vi "Lockin-4461 -Patrick -State.vi"(10 "IV Curve Mode":bool, 11 "Channels: AO":T6={"AO amp (V)"=[0.01, 0.0, 0.0, 0.0, 0.0, 0.0, 0.0, 0.0], "AO DC (V)"=[0.0, 0.0, 0.0, 0.0, 0.0, 0.0, 0.0, 0.0], "AO f (Hz)"=[13.1, 13.0, 13.0, 13.0, 13.0, 13.0, 13.0, 13.0], "AO phi (deg)"=[0.0, 0.0, 0.0, 0.0, 0.0, 0.0, 0.0, 0.0], "function"=[enum."Sine Wave", enum."Sine Wave", enum."Sine Wave", enum."Sine Wave", enum."Sine Wave", enum."Sine Wave", enum."Sine Wave", enum."Sine Wave"]} {"AO f (Hz)" min=0.001 max=10000.0; "AO DC (V)" format="%#_6p"; "AO amp (V)" format="%#_6p"}) -> ()   [LabVIEW 2016]
uses:
  Typedefs/AO-cluster.ctl
  Typedefs/AO_Amp-array.ctl
  Typedefs/AO_DC-array.ctl
  Typedefs/AO_f-array.ctl
  Typedefs/AO_phi-array.ctl
  Typedefs/Function-array.ctl
  Typedefs/Function-enum.ctl
  Typedefs/REF-cluster.ctl
  Typedefs/REF_f-array.ctl
  Typedefs/REF_phi-array.ctl
  Typedefs/AO.config-cluster.ctl
  Typedefs/AI.config-cluster.ctl
  Typedefs/AI.coupling-enum.ctl
  <vilib>/Analysis/4window.llb/windowTd.ctl
  <vilib>/measure/maspectr.llb/Power Spectrum and PSD Export Mode.ctl
  <vilib>/Utility/error.llb/DialogType.ctl
  <vilib>/Analysis/baseanly.llb/Mean (DBL).vi
  <userlib>/_OpenG.lib/array/array.llb/Empty 1D Array (Variant)__ogtk.vi
  <vilib>/Platform/browser.llb/Open URL in Default Browser (string).vi
  <userlib>/_OpenG.lib/error/error.llb/Filter Error Codes (Array)__ogtk.vi
  <userlib>/_OpenG.lib/array/array.llb/Empty 1D Array (DBL)__ogtk.vi
  <vilib>/measure/maspectr.llb/FFT Power Spectrum and PSD for N Chan.vi
  <vilib>/Waveform/WDTOps.llb/WDT Waveform to XY Pairs DBL.vi
  <vilib>/measure/NI_MAPro.lvlib
  <vilib>/Analysis/NI_AALBase.lvlib
  <vilib>/Utility/config.llb/NI_LVConfig.lvlib
  <vilib>/Analysis/NI_AALPro.lvlib
panel:
  in  "Tab Control 3":enum32{"Page 1"}(tab)
  in  "Bug":bool
  in  "Trigger":bool
  in  "Notes":string
  in  "Path":path=path "C:/Data/lockin"
  in  "EXIT":bool
  in  "RESET":bool
  in  "Save Data":bool
  out "X or R":dbl=-1.5674776385045113e-05 caption="X or R: Current (A) or Voltage (V)" format="%#.3p"
  out "Y or Theta":dbl=0.0006969030734106954 caption="Y or Theta: Current (A) or Voltage (V)" format="%.3p"
  in  "Display":enum16{"X and Y", "R and Theta"}(ring)
  in  "Channel":dbl min=0.0 max=7.0 step=1.0
  in  "Remote Mode":bool
  out "time and date":string="18:32:49.6   2017-07-28"
  out "DAQ mode string":string="None"
  out "time since trigger":dbl
  in  "mean":dbl[](array[numeric])=[0.0020212134088697844, -0.0038683061420776745, -0.0017577206979397751, -6.13137174522516e-05, -0.0025607955795279433, -0.0022408587829792284, 0.0003178164150233449, -0.0028469064949645513]
  in  "Tab Control 2":T1(tab)
  in  "Output signals?":bool=TRUE
  out "Signals Graph":waveform(dbl)[](graph)
  out "Reference Graph":waveform(dbl)[](graph)
  in  "decimate graph":i32=1
  in  "Display n?":bool=TRUE
  out "Display X (or R)":waveform(dbl)[](graph)=[{"t0"=timestamp(3584125969.6966953 s since 1904-01-01), "dt"=1.0, "Y"=[-1.5674776385045113e-05]}, {"t0"=timestamp(3584125969.6966953 s since 1904-01-01), "dt"=1.0, "Y"=[-8.70673776379909e-05]}, {"t0"=timestamp(3584125969.6966953 s since 1904-01-01), "dt"=1.0, "Y"=[-2.1693329226816633e-05]}, {"t0"=timestamp(3584125969.6966953 s since 1904-01-01), "dt"=1.0, "Y"=[-8.095080721838651e-05]}, {"t0"=timestamp(3584125969.6966953 s since 1904-01-01), "dt"=1.0, "Y"=[-9.220716518858501e-05]}, {"t0"=timestamp(3584125969.6966953 s since 1904-01-01), "dt"=1.0, "Y"=[-8.659365208742522e-05]}, {"t0"=timestamp(3584125969.6966953 s since 1904-01-01), "dt"=1.0, "Y"=[-0.0001111506406949471]}, {"t0"=timestamp(3584125969.6966953 s since 1904-01-01), "dt"=1.0, "Y"=[2.9050024564198337e-06]}]
  out "Display Y (or Theta)":waveform(dbl)[](graph)=[{"t0"=timestamp(3584125969.6966953 s since 1904-01-01), "dt"=1.0, "Y"=[0.0006969030734106954]}, {"t0"=timestamp(3584125969.6966953 s since 1904-01-01), "dt"=1.0, "Y"=[5.552511744346625e-05]}, {"t0"=timestamp(3584125969.6966953 s since 1904-01-01), "dt"=1.0, "Y"=[0.0001768914126496754]}, {"t0"=timestamp(3584125969.6966953 s since 1904-01-01), "dt"=1.0, "Y"=[3.781436113329896e-05]}, {"t0"=timestamp(3584125969.6966953 s since 1904-01-01), "dt"=1.0, "Y"=[-0.00011680861026454419]}, {"t0"=timestamp(3584125969.6966953 s since 1904-01-01), "dt"=1.0, "Y"=[-9.443651807610673e-05]}, {"t0"=timestamp(3584125969.6966953 s since 1904-01-01), "dt"=1.0, "Y"=[8.143626032195178e-05]}, {"t0"=timestamp(3584125969.6966953 s since 1904-01-01), "dt"=1.0, "Y"=[-0.0003099144140816687]}]
  out "XY Graph":cluster{dbl[], dbl[]}[](graph)=[{[0.0, -1.5674776385045113e-05], [0.0, 0.0006969030734106954]}, {[0.0, -8.70673776379909e-05], [0.0, 5.552511744346625e-05]}, {[0.0, -2.1693329226816633e-05], [0.0, 0.0001768914126496754]}, {[0.0, -8.095080721838651e-05], [0.0, 3.781436113329896e-05]}, {[0.0, -9.220716518858501e-05], [0.0, -0.00011680861026454419]}, {[0.0, -8.659365208742522e-05], [0.0, -9.443651807610673e-05]}, {[0.0, -0.0001111506406949471], [0.0, 8.143626032195178e-05]}, {[0.0, 2.9050024564198337e-06], [0.0, -0.0003099144140816687]}]
  out "Results\n(X, Y, R, Theta, mean)":dbl[][](array[numeric])=[[-1.5674776385045113e-05, 0.0006969030734106954, 0.000697079330022053, 91.28848209297018, 0.0020212134088697844], [-8.70673776379909e-05, 5.552511744346625e-05, 0.00010326551658645415, 147.4732893773882, -0.0038683061420776745], [-2.1693329226816633e-05, 0.0001768914126496754, 0.000178216644570985, 96.99163795294015, -0.0017577206979397751], [-8.095080721838651e-05, 3.781436113329896e-05, 8.934740677394016e-05, 154.96142087956403, -6.13137174522516e-05], [-9.220716518858501e-05, -0.00011680861026454419, 0.00014881670855132224, -128.28709336414173, -0.0025607955795279433], [-8.659365208742522e-05, -9.443651807610673e-05, 0.00012812773520271432, -132.51929584201363, -0.0022408587829792284], [-0.0001111506406949471, 8.143626032195178e-05, 0.0001377908902000489, 143.77104596378203, 0.0003178164150233449], [2.9050024564198337e-06, -0.0003099144140816687, 0.0003099280288951869, -89.46295009810324, -0.0028469064949645513]] format="%#_3p"
  out "PS Chart":dbl[][](graph)=[[-1105.6899114588311, -1143.9798102016132, -1120.3260349628486, -1104.2479960602075, -1135.3349531393583, -1128.801716551488, -1154.426424169608, -1125.1608260528487]]
  out "PS dB":cluster{"f0":dbl, "df":dbl, "magnitude":dbl[]}[](graph)
  in  "window":T2=1 items=["Rectangle"=0, "Hanning"=1, "Hamming"=2, "Blackman-Harris"=3, "Exact Blackman"=4, "Blackman"=5, "Flat Top"=6, "4 Term B-Harris "=7, "7 Term B-Harris"=8, "Low Sidelobe"=9, "Blackman Nuttall"=11, "Triangle"=30, "Bartlett-Hanning"=31, "Bohman"=32, "Parzen"=33, "Welch"=34, "Kaiser"=60, "Dolph-Chebyshev"=61, "Gaussian"=62]
  in  "averaging parameters":T3={"averaging mode"=enum."RMS averaging", "weighting mode"=enum."Exponential", "number of averages"=10} {"number of averages" min=1}
  in  "restart averaging (F)":bool
  in  "export mode":T4 items=["Power Spectrum", "Power Spectral Density"]
  in  "window parameter":dbl=nan
  out "averages\ncompleted":dbl=2.0
  out "averaging done":bool
  in  "Tab Control":T5(tab)
  in  "...............reset REF":bool
  in  "............zero offset":bool
  in  "....measure offset":bool
  in  "............all  f same":bool
  in  "..........reset signal":bool
  in  "60 Hz prefilter":bool
  in  "LP prefilter":bool
  in  "LP cutoff (Hz)":dbl=30.0
  in  "Channels: Lockin":T13={"REF f (Hz)"=[13.0], "REF phi (deg)"=[0.0, 0.0, 0.0, 0.0, 0.0, 0.0, 0.0, 0.0]} {"REF phi (deg)" format="%#_3g"}
  in  "D":dbl=0.019999999999999997 format="%.2f"
  in  "I":dbl=0.6 format="%.2f"
  in  "P":dbl=0.5 format="%.2f"
  in  "autophase?\n(experimental)":bool
  out "filter fC (Hz)":dbl=0.5305164769729844
  in  "TC (s)":dbl=0.3 format="%#_6p"
  in  "order":i32=2
  in  "save config":bool
  in  "load config":bool
  in  "Instrument":u16(ring) items=["SIMULATE", "CF900", "DR200", "MNK", "PPMS1", "PPMS2", "THz1", "THz2"]
  in  "AO Configuration":T16[](array[typedef])
  in  "AI Configuration":T17[](array[typedef])
  in  "#s":i32=15630
  in  "Fs":i32=204753
  in  "auto size":bool=TRUE
  in  "decimating factor":i32=1
  in  "AI Buffer Size (S)":i32=100
  out "dt":dbl=4.883933324542254e-06 format="%#_6p"
  in  "frequency multiplier":dbl=100000.0 format="%#_13g"
  out "sampling info":cluster{"Fs":i32, "#s":i32}={"Fs"=4000, "#s"=10000}
  in  "DAQ Type":enum16{"None", "USB 4431", "PXI 446x"}(ring)
  in  "Amplifiers":enum16{"None", "Krohn Hite", "Femto"}(ring)
  out "Current State":string="Exit"
  out "State History":string="4461: PHASE\r4461: LOCKIN\rMacro: Continuous\r4461: READ WRITE\r4461: FILTER\r4461: PHASE\r4461: LOCKIN\r4461: STOP TASKS\rMacro: Exit\rData: Cleanup\rExit"
  in  "offsets":dbl[](array[numeric])=[0.0, 0.0, 0.0, 0.0, 0.0, 0.0, 0.0, 0.0] format="%#.2p"
  in  "Gain":dbl[](array[numeric])=[1.0, 1.0, 1.0, 1.0, 1.0, 1.0, 1.0, 1.0]
  out "phase log":dbl[](array[numeric])=[0.0, 272.06106870229246, 272.06106870229246, 272.06106870229246, 272.06106870229246, 272.06106870229246, 272.06106870229246, 272.06106870229246] format="%.1f"
  out "AI tasks":i32
  out "AO tasks":i32
  out "error":errorcluster
  in  "Check Calibration":bool
  in  "Self Calibrate":bool
  out "Cal Info":T19(array[cluster])
  # "´"
  # "Multichannel Lockin v2017/10/09 v2.4.4"
  # "plot 0    = AI0 f0\nplot 1    = Ai1 f0\n...\nplot N-1  = AIN f0\n\nplot N    = AI0 f1\nplot N+1  = AI1 f1\n..."
  # "AO Settings"
  # "Lockin Settings"
  # "prefilters"
  # "lockin filter"
  # "autophase"
  # "0"
  # "1"
  # "2"
  # "3"
  # "4"
  # "5"
  # "6"
  # "7"
  # "configuration"
  # "sampling"
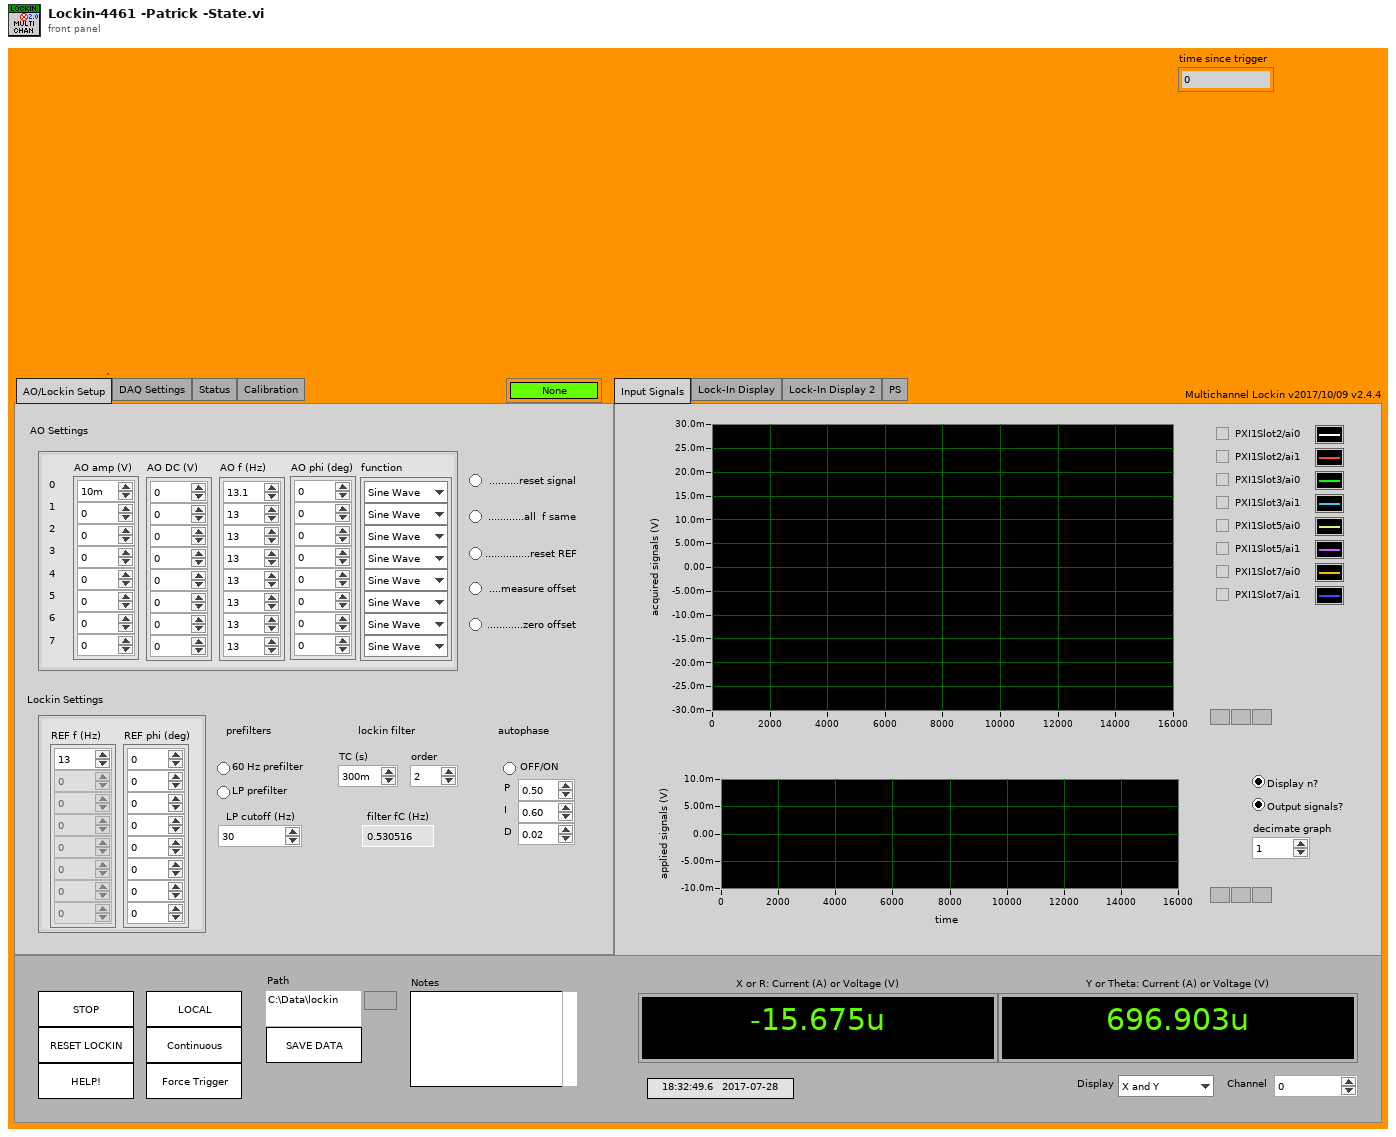
[diagram p1: front panel]
types:
  T1 = enum32{"Input Signals", "Lock-In Display", "Lock-In Display 2", "PS"}
  T2 = typedef "NI_AALPro.lvlib/windowTd.ctl" = u32
  T3 = cluster{"averaging mode":enum16{"No averaging", "Vector averaging", "RMS averaging", "Peak hold"}, "weighting mode":enum16{"Linear", "Exponential"}, "number of averages":u32}
  T4 = typedef "NI_MAPro.lvlib/Power Spectrum and PSD Export Mode.ctl" = u16
  T5 = enum32{"AO/Lockin Setup", "DAQ Settings", "Status", "Calibration"}
  T6 = typedef "AO-cluster.ctl" = cluster{"AO amp (V)":T7, "AO DC (V)":T8, "AO f (Hz)":T9, "AO phi (deg)":T10, "function":T11}
  T7 = typedef "AO_Amp-array.ctl" = dbl[]
  T8 = typedef "AO_DC-array.ctl" = dbl[]
  T9 = typedef "AO_f-array.ctl" = dbl[]
  T10 = typedef "AO_phi-array.ctl" = dbl[]
  T11 = typedef "Function-array.ctl" = T12[]
  T12 = typedef "Function-enum.ctl" = enum16{"Sine Wave", "Triangle Wave", "Square Wave", "Sawtooth Wave"}
  T13 = typedef "REF-cluster.ctl" = cluster{"REF f (Hz)":T14, "REF phi (deg)":T15}
  T14 = typedef "REF_f-array.ctl" = dbl[]
  T15 = typedef "REF_phi-array.ctl" = dbl[]
  T16 = typedef "AO.config-cluster.ctl" = cluster{"Output physical channels":tag, "AO. Max":dbl, "AO.Min":dbl}
  T17 = typedef "AI.config-cluster.ctl" = cluster{"AI.Coupling":T18, "AI.Max":dbl, "AI.Min":dbl, "Input physical channels":tag}
  T18 = typedef "AI.coupling-enum.ctl" = enum16{"AC", "DC", "GND"}
  T19 = cluster{tag, "SelfCal.LastDate/Time":timestamp, "SelfCal.LastTemp":dbl, "DevTemp":dbl, "calibration due?":bool}[]
  T20 = enum32{"invalid app kind", "Development System", "Run Time System", "Student Edition", "Embedded LabVIEW", "Evaluation", "Custom"}
  T21 = enum32{"Invalid", "Standard", "Closed", "Hidden", "Minimized", "Maximized"}
  T22 = cluster{"REF f (Hz)":dbl[], "REF phi (deg)":dbl[]}
  T23 = cluster{"AO amp (V)":dbl[], "AO DC (V)":dbl[], "AO f (Hz)":dbl[], "AO phi (deg)":dbl[], "function":enum16{"Sine Wave", "Triangle Wave", "Square Wave", "Sawtooth Wave"}[]}
  T24 = cluster{"Core":cluster{"Current VI Reference":refnum<vi>, "Close Panel on Exit?":bool}, "Error":bool, "Your string data":string, "AI task":refnum<k21>[], "AO task":refnum<k21>[], "Input Signals":waveform(dbl)[], "Ouput Signals":waveform(dbl)[], "REF":waveform(dbl)[], "sampling info":cluster{"Fs":dbl, "#s":dbl}, "Tasks":string[], "to":i32}
  T25 = typedef "DialogType.ctl" = u16
  T26 = cluster{"Current VI Reference":refnum<vi>, "Close Panel on Exit?":bool}
  T27 = cluster{"Output physical channels":tag, "AO. Max":dbl, "AO.Min":dbl}[]
  T28 = cluster{"AI.Coupling":enum16{"AC", "DC", "GND"}, "AI.Max":dbl, "AI.Min":dbl, "Input physical channels":tag}[]
  T29 = cluster{tag, "SelfCal.LastDate/Time":timestamp, "SelfCal.LastTemp":dbl, "DevTemp":dbl, "recalibrate?":bool}[]
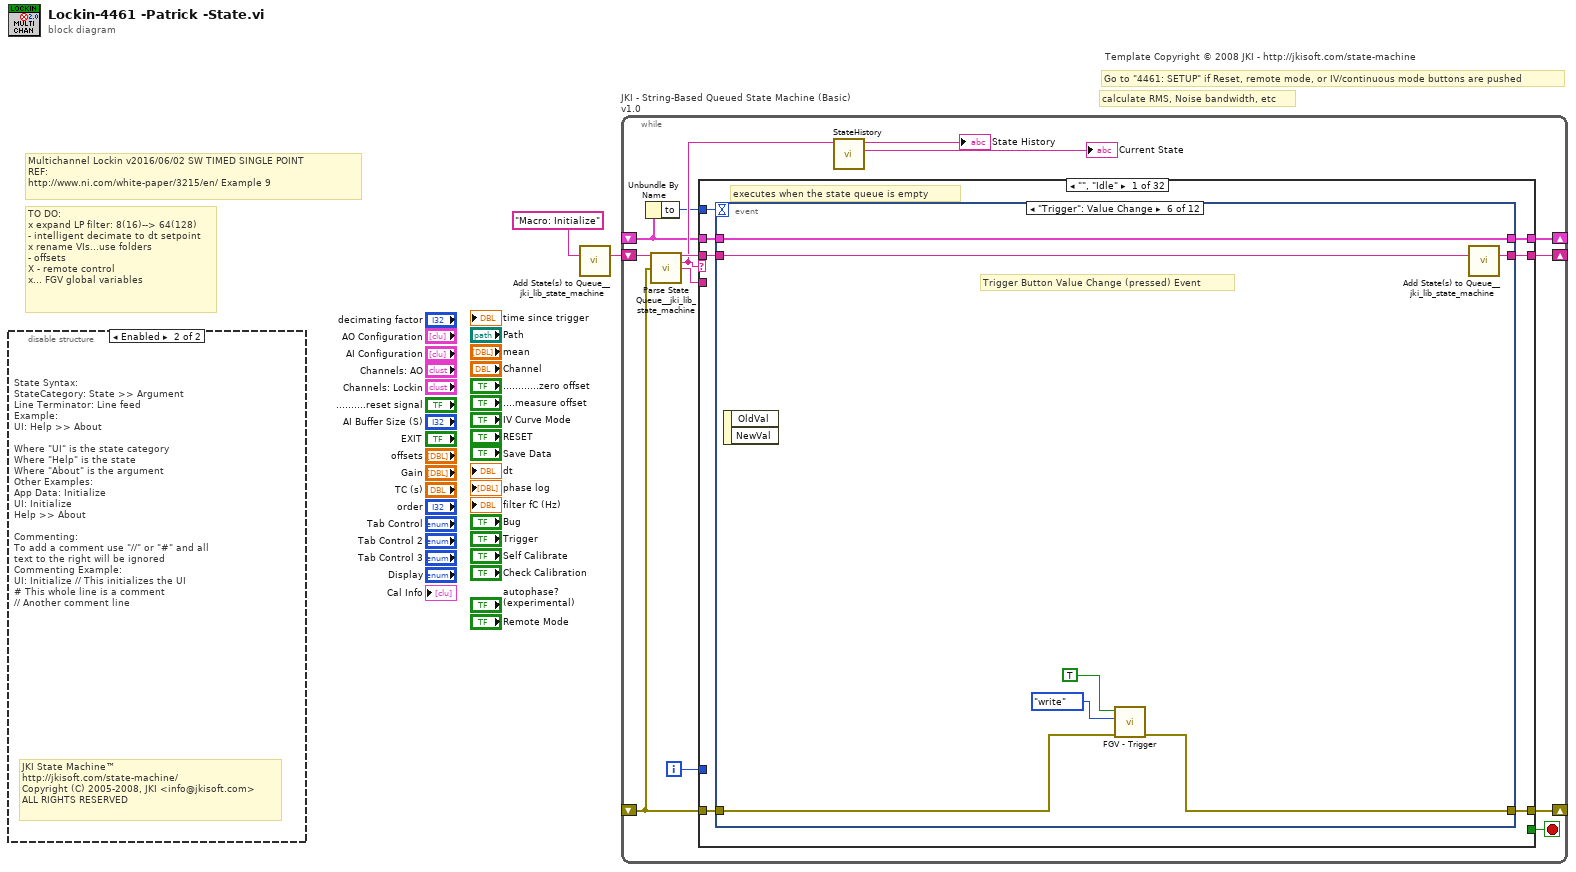
[diagram p0: block diagram]
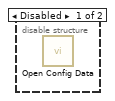
[diagram p2: hidden frame]
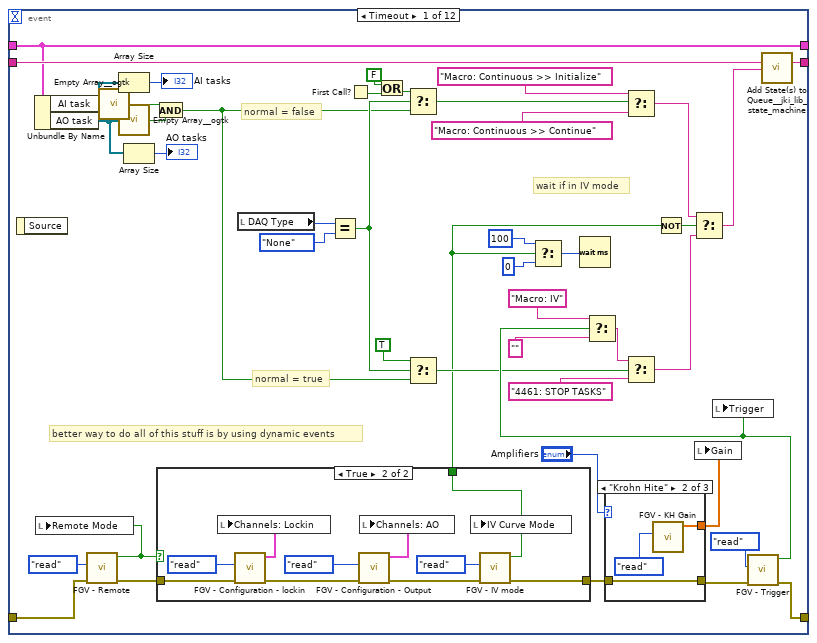
[diagram p3: hidden frame]
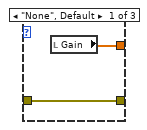
[diagram p4: hidden frame]
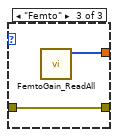
[diagram p5: hidden frame]
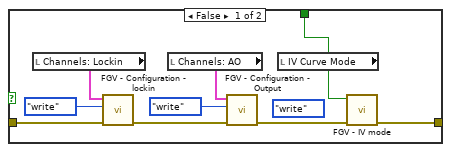
[diagram p6: hidden frame]
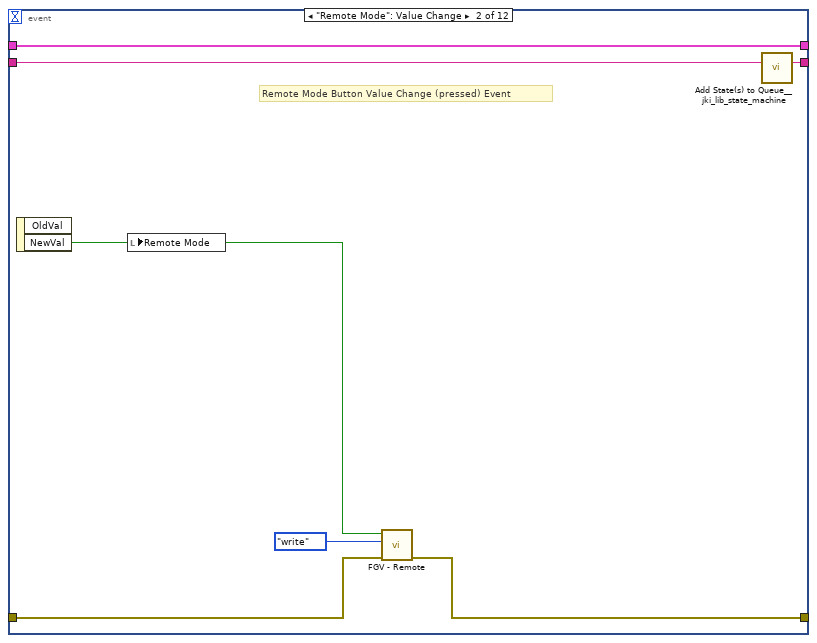
[diagram p7: hidden frame]
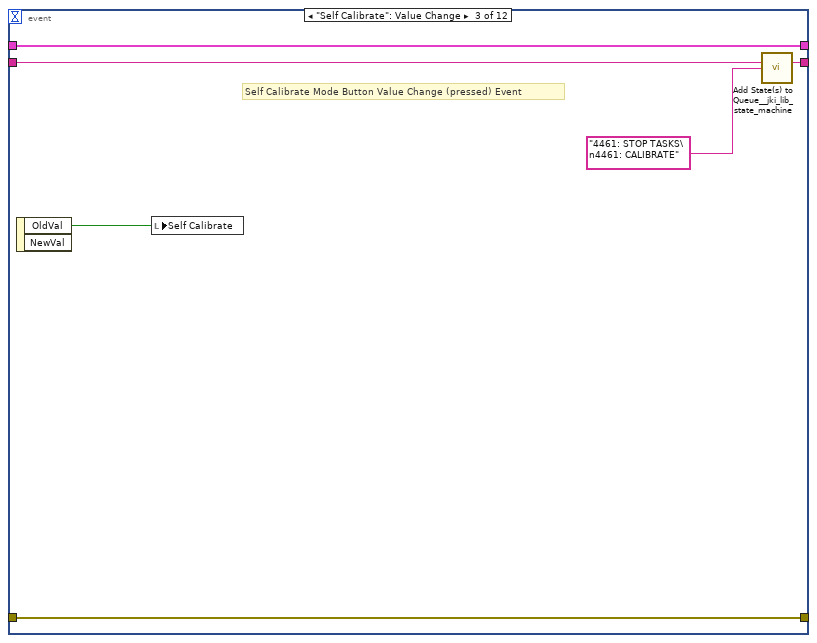
[diagram p8: hidden frame]
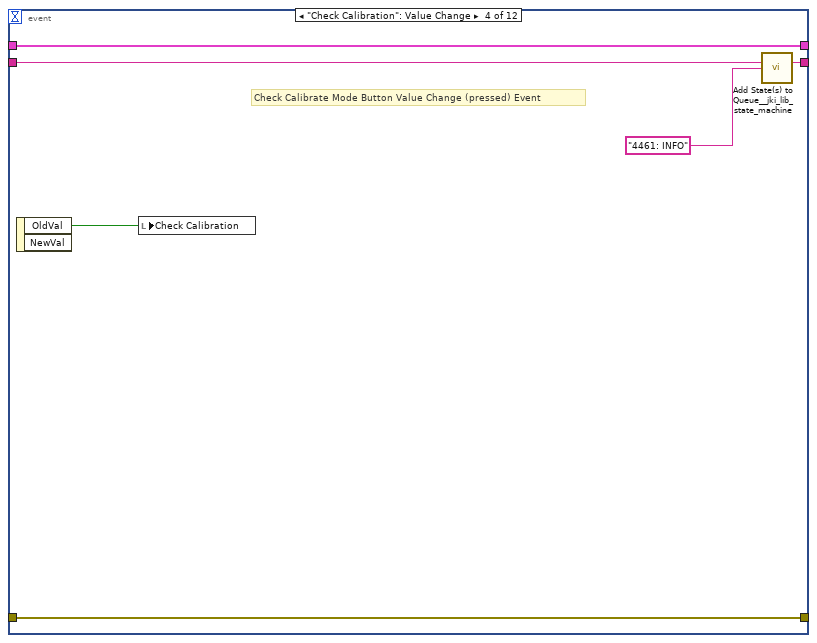
[diagram p9: hidden frame]
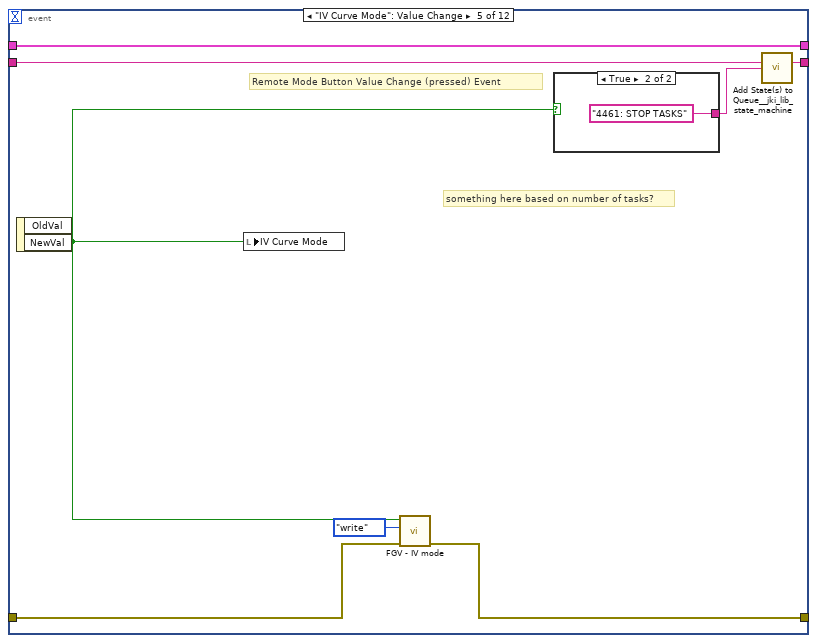
[diagram p10: hidden frame]
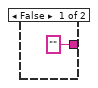
[diagram p11: hidden frame]
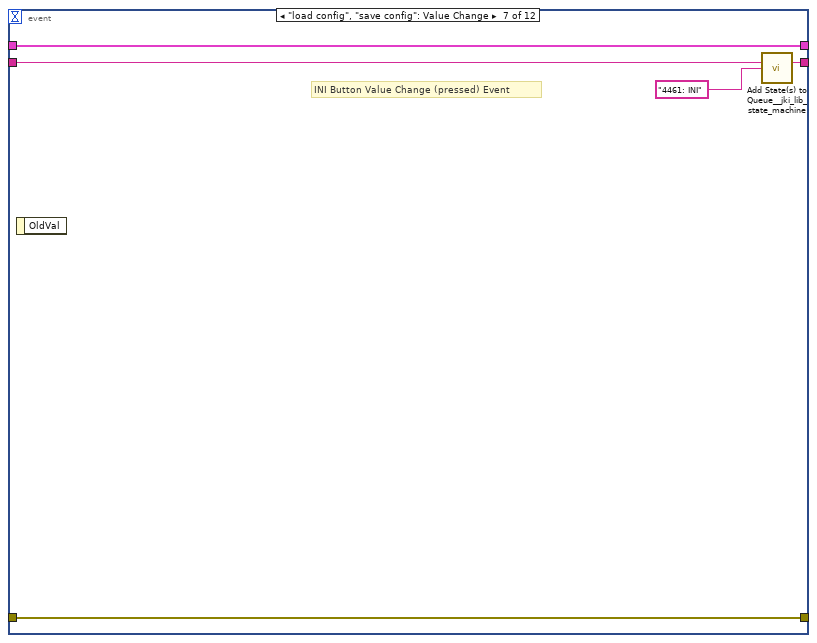
[diagram p12: hidden frame]
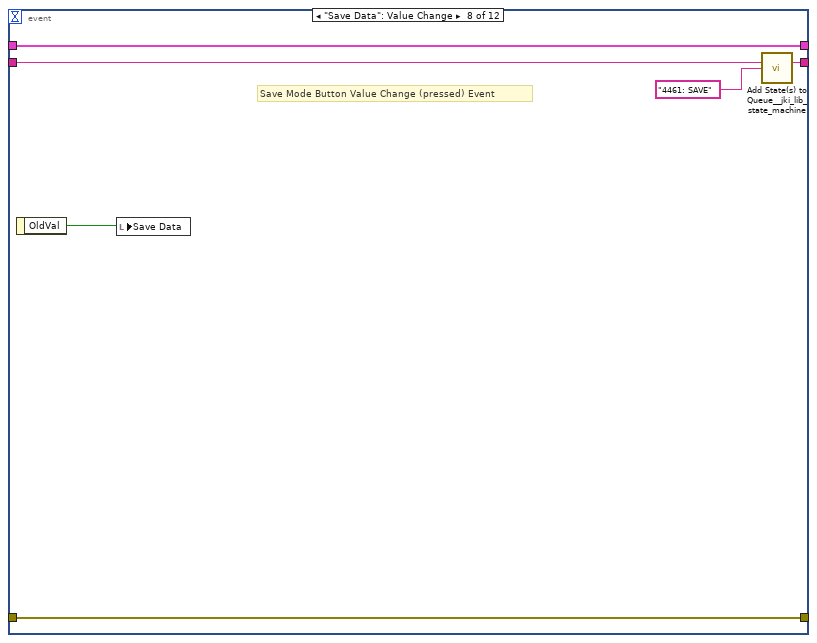
[diagram p13: hidden frame]
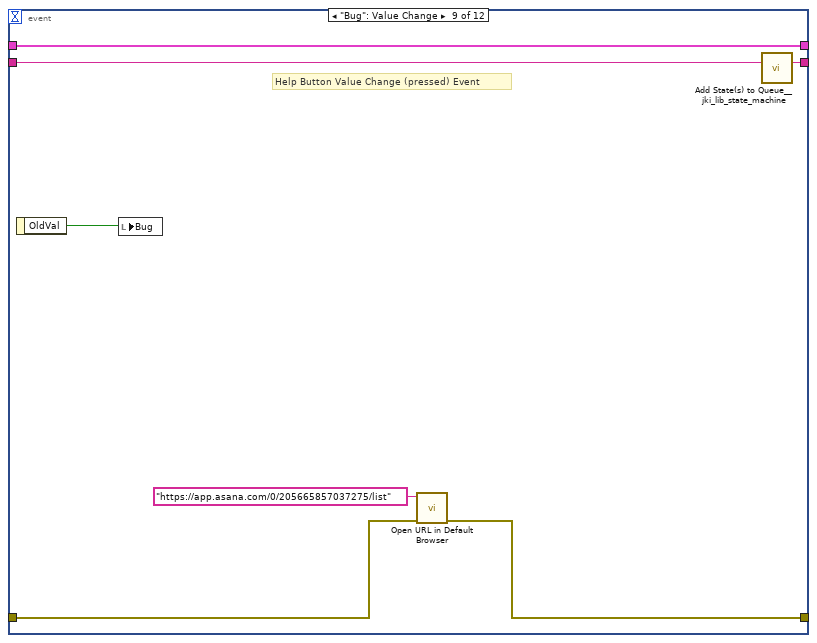
[diagram p14: hidden frame]
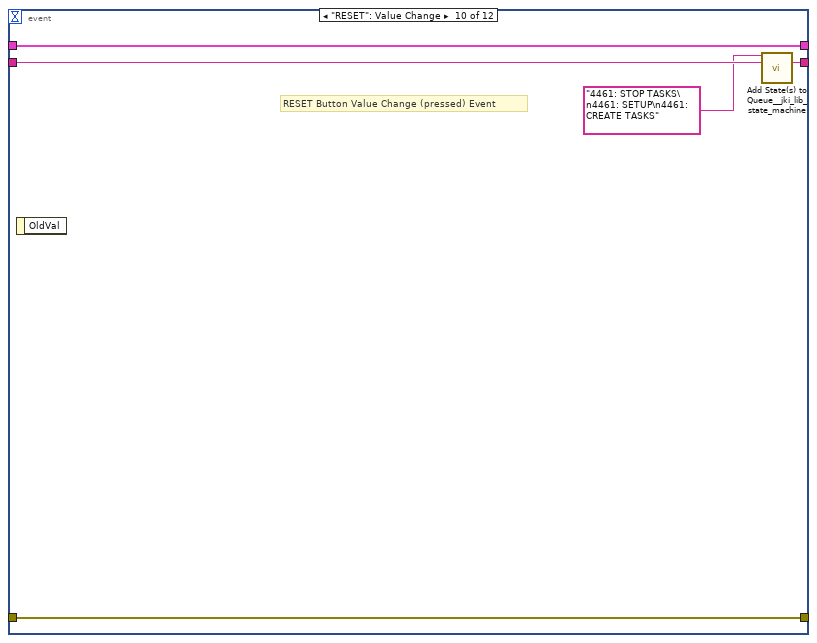
[diagram p15: hidden frame]
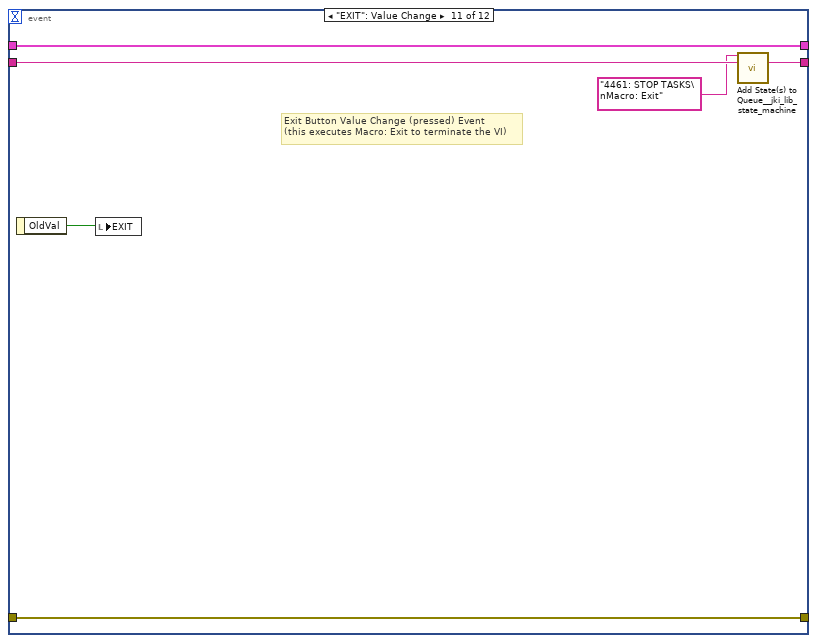
[diagram p16: hidden frame]
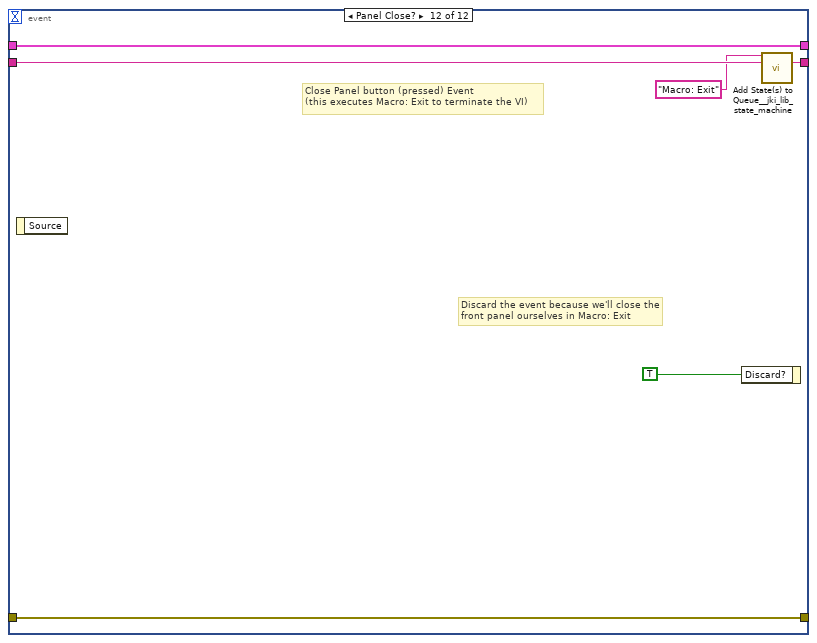
[diagram p17: hidden frame]
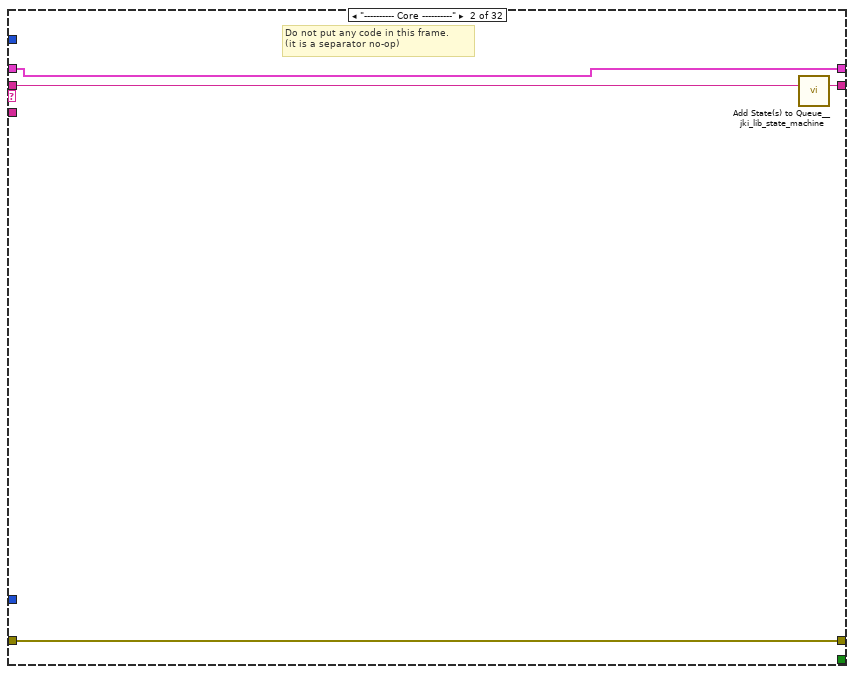
[diagram p18: hidden frame]
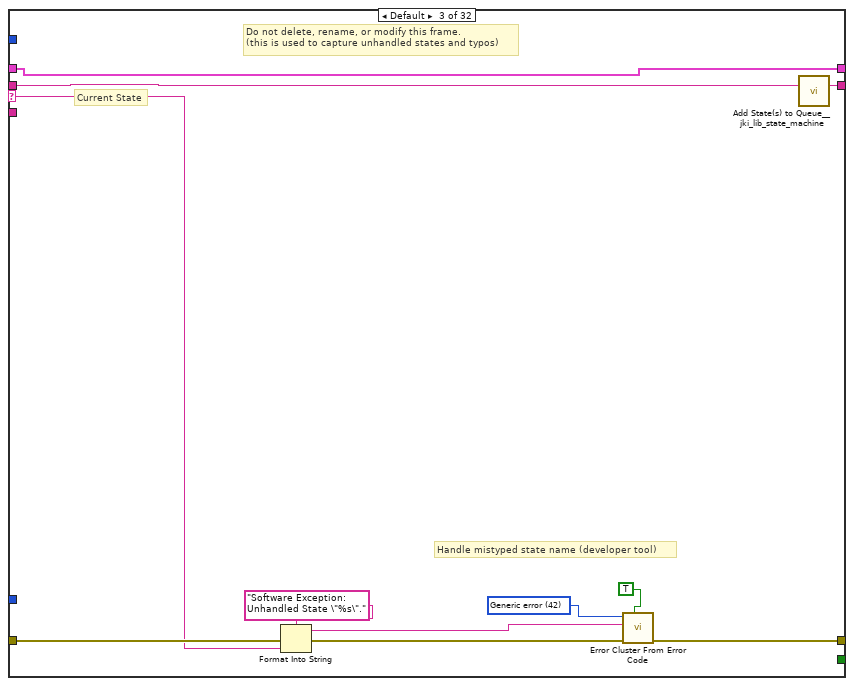
[diagram p19: hidden frame]
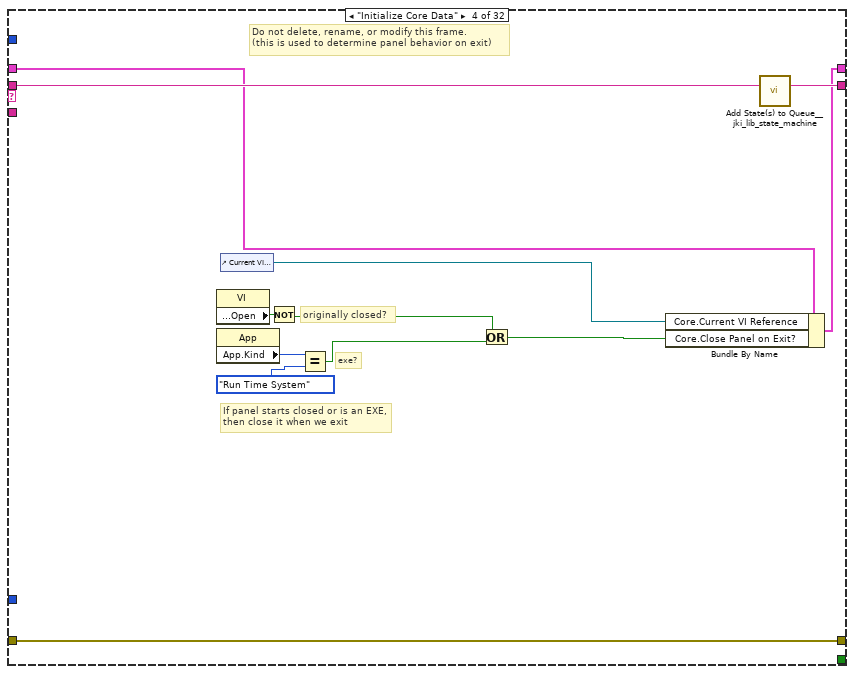
[diagram p20: hidden frame]
diagram:
  # "calculate RMS, Noise bandwidth, etc"
  # "Template Copyright © 2008 JKI - http://jkisoft.com/state-machine"
  # "Go to \"4461: SETUP\" if Reset, remote mode, or IV/continuous mode buttons are pushed"
  # "Multichannel Lockin v2016/06/02 SW TIMED SINGLE POINT\nREF:\nhttp://www.ni.com/white-paper/3215/en/ Example 9"
  # "TO DO:\nx expand LP filter: 8(16)--> 64(128)\n- intelligent decimate to dt setpoint\nx rename VIs...use folders\n- offsets\nX - remote control\nx... FGV global variables"
  n1 = disable-structure shown="Enabled" {
    frame Disabled {
      n2 = call <vilib>:"Open Config Data.vi"() -> ()  [unwired: 9 in, 3 out]
    }
    frame Enabled {
      # "JKI State Machine™\nhttp://jkisoft.com/state-machine/\nCopyright (C) 2005-2008, JKI <info@jkisoft.com>\nALL RIGHTS RESERVED"
      # "State Syntax:\nStateCategory: State >> Argument\nLine Terminator: Line feed\nExample:\nUI: Help >> About\n\nWhere \"UI\" is the state category\nWhere \"Help\" is the state\nWhere \"About\" is the argument\nOther Examples:\nApp Data: Initialize\nUI: Initialize\nHelp >> About\n\nCommenting:\nTo add a comment use \"//\" or \"#\" and all text to the right will be ignored\nCommenting Example:\nUI: Initialize // This initializes the UI\n# This whole line is a comment\n// Another comment line"
    }
  }
  n3 = call <vilib>:"Add State(s) to Queue__jki_lib_state_machine.vi"("State(s) in (\"\")"="Macro: Initialize") -> ("States Out"=w2:string)  [unwired: 14 in]
  n4 = while "JKI - String-Based Queued State Machine (Basic) v1.0" {
    shift-right: [w7] -> _
    shift-left: _ -> [w4]
    shift-right: [w15] -> _
    shift-left: _ -> [w8]
    shift-right: [w14] -> _
    shift-left: w2 -> [w9]
    i -> [w11]
    stop <- w13 stop-if-true
    n5 = Unbundle By Name(w4) -> ("to"=w3:i32)
    n6 = call <vilib>:"Parse State Queue__jki_lib_state_machine.vi"("State Queue"=w9, "Error In (no error)"=w8) -> ("Remaining States"=w12:string, "Current State"=w5:string, "Arguments"=w16:string)  [unwired: 11 in]
    n7 = case shown="\"\", \"Idle\"" w5 {
      selector: w5 -> [_ _ w169 _ _ _ _ _ _ _ _ _ _ _ _ _ _ _ _ _ _ _ _ _ _ _ _ _ _ _ _ _]
      tunnel: w16 -> [_ _ _ _ _ _ _ _ _ _ _ w256 w267 _ _ _ w309 _ _ _ _ _ _ _ _ _ _ _ _ _ _ _]
      tunnel: w4 -> [w21 w165 w171 w182 w197 w209 w212 _ w231 w237 w252 w255 w266 w294 w298 w303 w310 w316 w327 w336 w364 w414 w423 w436 w514 w565 w621 w686 w717 w765 w793 w841]
      tunnel: [w20 w166 w175 w188 errorcluster {"status"=FALSE, "code"=0, "source"=""} ("error out") w208 w213 w227 w232 w238 w246 w257 w265 w295 w300 w305 w311 w324 w328 w333 w366 w412 w419 w438 w522 w575 w610 w687 w719 w755 w794 w840] -> w15
      tunnel: w8 -> [w19 w166 w174 w188 w194 w208 w213 w227 w233 w238 w247 w258 w269 w295 w300 w305 w311 w324 w328 w334 w366 w413 w422 w442 w524 w578 w610 w687 w719 w754 w803 w840]
      tunnel: [w22 w167 w172 w190 w201 w210 w214 w229 w235 w239 w253 w259 w270 w296 w301 w306 w312 w325 w329 w338 w371 w417 w426 w448 w526 w585 w622 w685 w718 w766 w790 w838] -> w14
      tunnel: [_ _ _ _ _ TRUE _ _ _ _ _ _ _ _ _ _ _ _ _ _ _ _ _ _ _ _ _ _ _ _ _ _] -> w13
      tunnel: [w18 w165 w171 w189 w198 w209 w212 w228 w231 w237 w252 w255 w266 w294 w298 w303 w310 w316 w327 w336 w370 w414 w423 w443 w525 w584 w621 w686 w717 w765 w792 w841] -> w7
      tunnel: w3 -> [w17 _ _ _ _ _ _ _ _ _ _ _ _ _ _ _ _ _ _ _ _ _ _ _ _ _ _ _ _ _ _ _]
      tunnel: w12 -> [w23 w168 w173 w191 w202 w211 w215 w230 w236 w240 w254 w260 w271 w297 w302 w307 w313 w326 w330 w337 w372 w418 w427 w449 w527 w586 w623 w688 w720 w767 w804 w842]
      tunnel: w11 -> [_ _ _ _ _ _ _ _ _ _ _ _ _ _ _ _ _ _ _ _ _ _ _ _ _ _ _ _ _ _ _ _]
      frame "", "Idle" {
        # "executes when the state queue is empty"
        n8 = event shown="[5] \"Trigger\": Value Change" {
          selector: _ -> [_ _ _ _ _ _ _ _ _ _ _ _]
          dyn-events: _ -> [_ _ _ _ _ _ _ _ _ _ _ _]
          timeout: w17 -> [_ _ _ _ _ _ _ _ _ _ _ _]
          tunnel: w23 -> [w67 w100 w106 w112 w120 w129 w134 w140 w147 w152 w158 w164]
          tunnel: [w66 w99 w105 w111 w119 w128 w133 w139 w146 w151 w157 w163] -> w22
          tunnel: w21 -> [w56 w98 w104 w110 w118 w127 w132 w138 w145 w150 w155 w161]
          tunnel: [w57 w95 w103 w109 w115 w124 w130 w137 w142 w149 w156 w162] -> w20
          tunnel: w19 -> [w64 w96 w103 w109 w116 w125 w130 w137 w144 w149 w156 w162]
          tunnel: [w56 w98 w104 w110 w118 w127 w132 w138 w145 w150 w155 w161] -> w18
          event Timeout {
            # "better way to do all of this stuff is by using dynamic events"
            # "wait if in IV mode"
            # "normal = true"
            # "normal = false"
            n9 = event-data() -> ()  [unwired: 1 in, 1 out]
            n10 = Unbundle By Name(w56) -> ("AI task"=w51:refnum<k21>[], "AO task"=w49:refnum<k21>[])
            n11 = call "FGV - Remote.vi"("error in"=w64, "Function"=enum16{"write", "read"}."read") -> ("error out"=w62:errorcluster, "Remote Mode"=w59:bool)  [unwired: 4 in]
            n12 = local write "Remote Mode"(w59) -> ()
            n13 = call-poly <userlib>:"Empty Array__ogtk.vi"("Array"=w51) -> ("Empty Array?"=w55:bool)  [unwired: 8 in]
            n14 = Array Size(array=w51) -> (size(s)=→"AI tasks":i32)
            n15 = call-poly <userlib>:"Empty Array__ogtk.vi"("Array"=w49) -> ("Empty Array?"=w43:bool)  [unwired: 8 in]
            n16 = Array Size(array=w49) -> (size(s)=→"AO tasks":i32)
            n17 = And(x=w55, y=w43) -> (x .and. y?=w42:bool)
            n18 = case shown="True" w59 {
              tunnel: [w77 w87] -> w61
              tunnel: w62 -> [w79 w90]
              tunnel: [w75 w84] -> w25
              frame False {
                (unwired) enum16{"write", "read"}."write" ("Function")
                n19 = local read "Channels: Lockin"() -> (w80:T13)
                n20 = call "FGV - Configuration - lockin.vi"("error in"=w79, "Function"=enum16{"write", "read"}."write", "Channels: Lockin"=w80) -> ("error out"=w81:errorcluster)  [unwired: 3 in, 1 out]
                n21 = local read "Channels: AO"() -> (w76:T6)
                n22 = call "FGV - Configuration - Output.vi"("error in"=w81, "Function"=enum16{"write", "read"}."write", "Channels: AO"=w76) -> ("error out"=w78:errorcluster)  [unwired: 3 in, 1 out]
                n23 = local read "IV Curve Mode"() -> (w75:bool)
                n24 = call "FGV - IV mode.vi"("error in"=w78, "IV mode"=w75) -> ("error out"=w77:errorcluster)  [unwired: 4 in, 1 out]
              }
              frame True {
                n25 = call "FGV - Configuration - lockin.vi"("error in"=w90, "Function"=enum16{"write", "read"}."read") -> ("error out"=w91:errorcluster, "Channels: Lockin 2"=w89:T22)  [unwired: 4 in]
                n26 = local write "Channels: Lockin"(w89) -> ()
                n27 = call "FGV - Configuration - Output.vi"("error in"=w91, "Function"=enum16{"write", "read"}."read") -> ("error out"=w88:errorcluster, "Channels: AO 2"=w86:T23)  [unwired: 4 in]
                n28 = local write "Channels: AO"(w86) -> ()
                n29 = call "FGV - IV mode.vi"("error in"=w88, "Function"=enum16{"write", "read"}."read") -> ("error out"=w87:errorcluster, "IV mode"=w84:bool)  [unwired: 4 in]
                n30 = local write "IV Curve Mode"(w84) -> ()
              }
            }
            n31 = local read "DAQ Type"() -> (w53:enum16{"None", "USB 4431", "PXI 446x"})
            n32 = Equal?(x=w53, y=enum16{"None", "USB 4431", "PXI 446x"}."None" ("DAQ Type")) -> (x = y?=w45:bool)
            n33 = First Call?() -> (First Call?: T/F=w39:bool)
            n34 = Or(x=FALSE ("t"), y=w39) -> (x .or. y?=w40:bool)
            n35 = Select(t=w40, s=w45, f=w42) -> (s? t:f=w37:bool)
            n36 = Select(t=TRUE, s=w45, f=w42) -> (s? t:f=w34:bool)
            n37 = Select(t=u32 100 ("milliseconds to wait"), s=w25, f=u32 0 ("milliseconds to wait")) -> (s? t:f=w24:u32)
            n38 = Wait (ms)(milliseconds to wait=w24) -> ()  [unwired: 1 out]
            n39 = case shown="\"Krohn Hite\"" "Amplifiers" {
              tunnel: [w69 w72 w73] -> w58
              tunnel: [w68 w71 w74] -> w63
              tunnel: w61 -> [w69 w72 w73]
              frame "None", Default {
                n40 = local read "Gain"() -> (w68:dbl[])
              }
              frame "Krohn Hite" {
                n41 = call <userlib>:"FGV - KH Gain.vi"("Function"=enum16{"write", "read"}."read") -> ("Gains"=w71:dbl[])  [unwired: 5 in, 1 out]
              }
              frame "Femto" {
                n42 = call <userlib>:"FemtoGain_ReadAll.vi"() -> ("Femto Gains"=w74:i32[])  [unwired: 11 in]
              }
            }
            n43 = Select(t="Macro: Continuous >> Initialize" ("State(s) at Back (\"\")"), s=w37, f="Macro: Continuous >> Continue" ("State(s) at Back (\"\")")) -> (s? t:f=w36:string)
            n44 = Not(x=w25) -> (.not. x?=w54:bool)
            n45 = local write "Gain"(w63) -> ()
            n46 = call "FGV - Trigger.vi"("error in"=w58, "Function"=enum16{"write", "read"}."read") -> ("error out"=w57:errorcluster, "Trigger 2"=w46:bool)  [unwired: 4 in]
            n47 = Select(t="Macro: IV" ("State(s) at Back (\"\")"), s=w46, f="" ("State(s) at Back (\"\")")) -> (s? t:f=w29:string)
            n48 = Select(t=w29, s=w34, f="4461: STOP TASKS" ("State(s) at Back (\"\")")) -> (s? t:f=w33:string)
            n49 = Select(t=w36, s=w54, f=w33) -> (s? t:f=w41:string)
            n50 = local write "Trigger"(w46) -> ()
            n51 = call <vilib>:"Add State(s) to Queue__jki_lib_state_machine.vi"("State(s) in (\"\")"=w67, "State(s) at Back (\"\")"=w41) -> ("States Out"=w66:string)  [unwired: 13 in]
          }
          event "Remote Mode": Value Change {
            # "Remote Mode Button Value Change (pressed) Event"
            n52 = event-data() -> ("NewVal"=w94:bool)  [unwired: 1 in, 1 out]
            n53 = local write "Remote Mode"(w94) -> ()
            n54 = call "FGV - Remote.vi"("error in"=w96, "Function"=enum16{"write", "read"}."write", "Remote Mode"=w94) -> ("error out"=w95:errorcluster)  [unwired: 3 in, 1 out]
            n55 = call <vilib>:"Add State(s) to Queue__jki_lib_state_machine.vi"("State(s) in (\"\")"=w100) -> ("States Out"=w99:string)  [unwired: 14 in]
          }
          event "Self Calibrate": Value Change {
            # "Self Calibrate Mode Button Value Change (pressed) Event"
            n56 = event-data() -> ("OldVal"=w101:bool)  [unwired: 1 in, 1 out]
            n57 = local write "Self Calibrate"(w101) -> ()
            n58 = call <vilib>:"Add State(s) to Queue__jki_lib_state_machine.vi"("State(s) in (\"\")"=w106, "State(s) at Back (\"\")"="4461: STOP TASKS\n4461: CALIBRATE" ("State(s) at Back (\"\")")) -> ("States Out"=w105:string)  [unwired: 13 in]
          }
          event "Check Calibration": Value Change {
            # "Check Calibrate Mode Button Value Change (pressed) Event"
            n59 = event-data() -> ("OldVal"=w107:bool)  [unwired: 1 in, 1 out]
            n60 = local write "Check Calibration"(w107) -> ()
            n61 = call <vilib>:"Add State(s) to Queue__jki_lib_state_machine.vi"("State(s) in (\"\")"=w112, "State(s) at Back (\"\")"="4461: INFO" ("State(s) at Back (\"\")")) -> ("States Out"=w111:string)  [unwired: 13 in]
          }
          event "IV Curve Mode": Value Change {
            # "something here based on number of tasks?"
            # "Remote Mode Button Value Change (pressed) Event"
            n62 = event-data() -> ("NewVal"=w113:bool)  [unwired: 1 in, 1 out]
            n63 = local write "IV Curve Mode"(w113) -> ()
            n64 = call "FGV - IV mode.vi"("error in"=w116, "Function"=enum16{"write", "read"}."write", "IV mode"=w113) -> ("error out"=w115:errorcluster)  [unwired: 3 in, 1 out]
            n65 = case shown="True" w113 {
              tunnel: ["" ("State(s) at Back (\"\")") "4461: STOP TASKS" ("State(s) at Back (\"\")")] -> w114
              frame False {
              }
              frame True {
              }
            }
            n66 = call <vilib>:"Add State(s) to Queue__jki_lib_state_machine.vi"("State(s) in (\"\")"=w120, "State(s) at Back (\"\")"=w114) -> ("States Out"=w119:string)  [unwired: 13 in]
          }
          event "Trigger": Value Change {
            # "Trigger Button Value Change (pressed) Event"
            n67 = event-data() -> ()  [unwired: 1 in, 2 out]
            n68 = call "FGV - Trigger.vi"("error in"=w125, "Function"=enum16{"write", "read"}."write", "Trigger"=TRUE) -> ("error out"=w124:errorcluster)  [unwired: 3 in, 1 out]
            n69 = call <vilib>:"Add State(s) to Queue__jki_lib_state_machine.vi"("State(s) in (\"\")"=w129) -> ("States Out"=w128:string)  [unwired: 14 in]
          }
          event "load config", "save config": Value Change {
            # "INI Button Value Change (pressed) Event"
            n70 = event-data() -> ()  [unwired: 1 in, 1 out]
            n71 = call <vilib>:"Add State(s) to Queue__jki_lib_state_machine.vi"("State(s) in (\"\")"=w134, "State(s) at Back (\"\")"="4461: INI") -> ("States Out"=w133:string)  [unwired: 13 in]
          }
          event "Save Data": Value Change {
            # "Save Mode Button Value Change (pressed) Event"
            n72 = event-data() -> ("OldVal"=w135:bool)  [unwired: 1 in]
            n73 = local write "Save Data"(w135) -> ()
            n74 = call <vilib>:"Add State(s) to Queue__jki_lib_state_machine.vi"("State(s) in (\"\")"=w140, "State(s) at Back (\"\")"="4461: SAVE") -> ("States Out"=w139:string)  [unwired: 13 in]
          }
          event "Bug": Value Change {
            # "Help Button Value Change (pressed) Event"
            n75 = event-data() -> ("OldVal"=w141:bool)  [unwired: 1 in]
            n76 = local write "Bug"(w141) -> ()
            n77 = call-poly <vilib>:"Open URL in Default Browser.vi"("error in (no error)"=w144, "URL"="https://app.asana.com/0/205665857037275/list") -> ("error out"=w142:errorcluster)  [unwired: 4 in, 1 out]
            n78 = call <vilib>:"Add State(s) to Queue__jki_lib_state_machine.vi"("State(s) in (\"\")"=w147) -> ("States Out"=w146:string)  [unwired: 14 in]
          }
          event "RESET": Value Change {
            # "RESET Button Value Change (pressed) Event"
            n79 = event-data() -> ()  [unwired: 1 in, 1 out]
            n80 = call <vilib>:"Add State(s) to Queue__jki_lib_state_machine.vi"("State(s) in Front (\"\")"="4461: STOP TASKS\n4461: SETUP\n4461: CREATE TASKS", "State(s) in (\"\")"=w152) -> ("States Out"=w151:string)  [unwired: 13 in]
          }
          event "EXIT": Value Change {
            # "Exit Button Value Change (pressed) Event\n(this executes Macro: Exit to terminate the VI)"
            n81 = event-data() -> ("OldVal"=w153:bool)  [unwired: 1 in]
            n82 = local write "EXIT"(w153) -> ()
            n83 = call <vilib>:"Add State(s) to Queue__jki_lib_state_machine.vi"("State(s) in Front (\"\")"="4461: STOP TASKS\nMacro: Exit", "State(s) in (\"\")"=w158) -> ("States Out"=w157:string)  [unwired: 13 in]
          }
          event Panel Close? {
            # "Discard the event because we'll close the front panel ourselves in Macro: Exit"
            # "Close Panel button (pressed) Event\n(this executes Macro: Exit to terminate the VI)"
            n84 = event-data() -> ()  [unwired: 1 in, 1 out]
            n85 = event-data("Discard?"=TRUE) -> ()  [unwired: 1 in, 1 out]
            n86 = call <vilib>:"Add State(s) to Queue__jki_lib_state_machine.vi"("State(s) in Front (\"\")"="Macro: Exit", "State(s) in (\"\")"=w164) -> ("States Out"=w163:string)  [unwired: 13 in]
          }
        }
      }
      frame "---------- Core ----------" {
        # "Do not put any code in this frame.\n(it is a separator no-op)"
        n87 = call <vilib>:"Add State(s) to Queue__jki_lib_state_machine.vi"("State(s) in (\"\")"=w168) -> ("States Out"=w167:string)  [unwired: 14 in]
      }
      frame Default {
        w178 = 42 items=["No error", "Argument error", "Memory is full", "Out of zone", "End of file", "File already open", "Generic file I/O error", "File not found", "File permission error", "Disk is full", "Duplicate path", "Too many files open", "System feature not enabled", "Resource file not found", "Cannot add resource", "Resource not found", "Image not found", "Image memory error", "Pen does not exist", "Config type invalid", "Config token not found", "Config parse error", "Config memory error", "Bad external code format", "Bad external code offset", "External code not present", "Null window", "Destroy window error", "Null menu", "Print aborted", "Bad print record", "Print driver error", "Windows error during printing", "Memory error during printing", "Print dialog error", "Generic print error", "Invalid device refnum", "Device not found", "Device parameter error", "Device unit error", "Cannot open device", "Device call aborted", "Generic error", "Cancelled by user", "Object ID too low", "Object ID too high", "Object not in heap", "Unknown heap", "Unknown object (invalid DefProc)", "Unknown object (DefProc not in table)", "Message out of range", "Invalid (null) method", "Unknown message", "Manager call not supported", "Bad address", "Network operation in progress", "Network operation timed out", "Connection is busy", "Network attribute not supported", "Network error", "Address in use", "System out of memory", "Connection aborted", "Connection refused", "Not connected", "Already connected", "Connection closed", "Initialization error (interapplication manager)", "Bad occurrence", "Wait on unbound occurrence handler", "Occurrence queue overflow", "Datalog type conflict", "Unused", "Unrecognized type (interapplication manager)", "Memory corrupt", "Failed to make temporary DLL", "Old CIN version", "Drag socket not found", "Failed to load drop-object", "Failed to register OLE object", "Failed to release OLE object", "Format specifier type mismatch", "Unknown format specifier", "Too few format specifiers", "Too many format specifiers", "Scan failed", "Newer CIN version", "Error converting to variant", "Runtime menu error", "Password tampered", "Variant attribute not found", "Incompatible variant data type", "Event data is not available", "Event Store is not present", "Occurrence is not found", "Event Queue is not created", "Event info is not available", "Refnum passed is NULL", "Error retrieving Class GUID", "Error retrieving CoClass GUID", "Error retrieving TypeLib GUID.", "Bad built application magic bytes.", "Specific driver is different from the specific driver associated with the Logical Name.", "There is no session opened to the class driver.", "Max Error", "MAX - Error with config objects", "MAX - Error loading configuration", "MAX - Group not supported"]
        # "Current State"
        # "Do not delete, rename, or modify this frame.\n(this is used to capture unhandled states and typos)"
        # "Handle mistyped state name (developer tool)"
        n88 = Format Into String(format string="Software Exception: Unhandled State \"%s\"." ("message"), error in=w174, w169) -> (resulting string=w177:string, error out=w176:errorcluster)  [unwired: 1 in]
        n89 = call <vilib>:"Error Cluster From Error Code.vi"("show call chain? (False)"=TRUE, "error in (no error)"=w176, "error message (\"\")"=w177, "error code (0)"=w178) -> ("error out"=w175:errorcluster)  [unwired: 5 in]
        n90 = call <vilib>:"Add State(s) to Queue__jki_lib_state_machine.vi"("State(s) in (\"\")"=w173) -> ("States Out"=w172:string)  [unwired: 14 in]
      }
      frame "Initialize Core Data" {
        # "Do not delete, rename, or modify this frame.\n(this is used to determine panel behavior on exit)"
        # "originally closed?"
        # "exe?"
        # "If panel starts closed or is an EXE, then close it when we exit"
        n91 = property class="VI"() -> ("Front Panel.Open"=w187:bool)  [unwired: 2 in, 2 out]
        n92 = property class="App"() -> ("App.Kind"=w186:T20)  [unwired: 2 in, 2 out]
        n93 = control-ref of="Current VI Reference"() -> (w180:refnum<vi>)
        n94 = Not(x=w187) -> (.not. x?=w184:bool)
        n95 = Equal?(x=w186, y=T20."Run Time System" ("Application:Kind")) -> (x = y?=w183:bool)
        n96 = Or(x=w184, y=w183) -> (x .or. y?=w181:bool)
        n97 = Bundle By Name(cluster=w182, "Core.Current VI Reference"=w180, "Core.Close Panel on Exit?"=w181) -> (w189:T24)
        n98 = call <vilib>:"Add State(s) to Queue__jki_lib_state_machine.vi"("State(s) in (\"\")"=w191) -> ("States Out"=w190:string)  [unwired: 14 in]
      }
      frame "Error Handler" {
        # "Handle any errors here.\nYou can also output any states to clean-up after errors occur"
        # "Clear error"
        n99 = Unbundle By Name(w197) -> ("Error"=w199:bool)
        n100 = Not(x=w199) -> (.not. x?=w192:bool)
        n101 = Bundle By Name(cluster=w197, "Error"=w192) -> (w198:T24)
        n102 = call-poly <userlib>:"Filter Error Codes__ogtk.vi"("Error In"=w194, "Error Codes to Filter"=i32[] [-200077]) -> ("Error Out"=w193:errorcluster)  [unwired: 7 in, 2 out]
        n103 = case shown="No Error" w193 {
          selector: w193 -> [_ w205]
          tunnel: ["4461: RESET" "Macro: Exit"] -> w196
          frame No Error {
          }
          frame Error {
            w206 = T25 1 items=["no dialog", "OK message", "continue or stop message", "OK message + warnings", "continue/stop + warnings"] ("type of dialog (OK msg:1)")
            # "Unhandled Error -- Display it"
            n104 = call <vilib>:"General Error Handler.vi"("type of dialog (OK msg:1)"=w206, "error in (no error)"=w205) -> ()  [unwired: 9 in, 5 out]
          }
        }
        n105 = call <vilib>:"Add State(s) to Queue__jki_lib_state_machine.vi"("State(s) in Front (\"\")"=w196, "State(s) in (\"\")"=w202) -> ("States Out"=w201:string)  [unwired: 13 in]
        "error" <- w194
      }
      frame "Exit" {
        # "Do not put any code in this frame.\n(No errors that occur here will be handled.)"
        n106 = call <vilib>:"Add State(s) to Queue__jki_lib_state_machine.vi"("State(s) in (\"\")"=w211) -> ("States Out"=w210:string)  [unwired: 14 in]
      }
      frame "---------- Data ----------" {
        # "Do not put any code in this frame.\n(It is a separator no-op. You can make a copy of this frame to create a new Data frame)"
        n107 = call <vilib>:"Add State(s) to Queue__jki_lib_state_machine.vi"("State(s) in (\"\")"=w215) -> ("States Out"=w214:string)  [unwired: 14 in]
      }
      frame "Data: Initialize" {
        w216 = 0  # to
        w217 = string[] []  # Tasks
        w218 = cluster{"Fs":dbl, "#s":dbl} {"Fs"=204800.0, "#s"=204800.0}  # sampling info
        w219 = waveform(dbl)[] []  # Ouput Signals
        w221 = waveform(dbl)[] []  # Input Signals
        w220 = waveform(dbl)[] []  # REF
        w222 = refnum<k21>[] []  # AO task
        w223 = refnum<k21>[] []  # AI task
        w224 = T26 {"Current VI Reference"=refnum, "Close Panel on Exit?"=FALSE}  # Core
        w226 = FALSE  # Error
        w225 = ""  # Your string data
        # "do not delete - used by framework"
        # "Expand Bundle to add new data elements to shift register data."
        # "Add new data here."
        # "Data names and types of shift register data are defined by this bundle."
        # "Initialize the shift-register data, here.\n(data names are defined by what you wire into the bundle function)"
        n108 = Bundle("Core"=w224, "Error"=w226, "Your string data"=w225, "AI task"=w223, "AO task"=w222, "Input Signals"=w221, "Ouput Signals"=w219, "REF"=w220, "sampling info"=w218, "Tasks"=w217, "to"=w216) -> (w228:T24)  [unwired: 1 in]
        n109 = call <vilib>:"Add State(s) to Queue__jki_lib_state_machine.vi"("State(s) in (\"\")"=w230) -> ("States Out"=w229:string)  [unwired: 14 in]
      }
      frame "Data: Cleanup" {
        # "Cleanup any data and references, here.\n(this is called automatically, by the Macro: Exit)"
        n110 = Unbundle By Name(w231) -> ("Core.Current VI Reference"=w234:refnum<vi>)
        n111 = Close Reference(reference=w234, error in (no error)=w233) -> (error out=w232:errorcluster)
        n112 = call <vilib>:"Add State(s) to Queue__jki_lib_state_machine.vi"("State(s) in (\"\")"=w236) -> ("States Out"=w235:string)  [unwired: 14 in]
      }
      frame "---------- UI ----------" {
        # "Do not put any code in this frame.\n(It is a separator no-op. You can make a copy of this frame to create a new UI frame)"
        n113 = call <vilib>:"Add State(s) to Queue__jki_lib_state_machine.vi"("State(s) in (\"\")"=w240) -> ("States Out"=w239:string)  [unwired: 14 in]
      }
      frame "UI: Initialize" {
        w242 = FALSE ("EXIT")
        w241 = waveform(dbl)[][] [] ("History Data")
        # "empty Display charts"
        # "Initialize the User Interface, here.\n(this is called automatically, by the Macro: Init)"
        n114 = property on="Display X (or R)" class="WaveformChart (strict)"("History Data"=w241) -> ()  [unwired: 2 in, 2 out]
        n115 = property on="Display Y (or Theta)" class="WaveformChart (strict)"("History Data"=w241) -> ()  [unwired: 2 in, 2 out]
        n116 = local write "error"(errorcluster {"status"=FALSE, "code"=0, "source"=""} ("error out")) -> ()
        n117 = local write "EXIT"(w242) -> ()
        n118 = local write "RESET"(w242) -> ()
        n119 = call "FGV - Remote.vi"("error in"=w247, "Function"=enum16{"write", "read"}."write", "Remote Mode"=w242) -> ("error out"=w248:errorcluster)  [unwired: 3 in, 1 out]
        n120 = local write "Bug"(w242) -> ()
        n121 = Initialize Array(1.0 ("element"), 8 ("dimension size")) -> (w243:dbl[])
        n122 = local write "Gain"(w243) -> ()
        n123 = local write "Remote Mode"(w242) -> ()
        n124 = call "FGV - Trigger.vi"("error in"=w248, "Function"=enum16{"write", "read"}."write", "Trigger"=w242) -> ("error out"=w246:errorcluster)  [unwired: 3 in, 1 out]
        n125 = local write "Trigger"(w242) -> ()
        n126 = call <vilib>:"Add State(s) to Queue__jki_lib_state_machine.vi"("State(s) in (\"\")"=w254) -> ("States Out"=w253:string)  [unwired: 14 in]
      }
      frame "UI: Cursor Set" {
        # "Argument"
        # "Set and Unset Cursor Busy.\n(Usage: \"UI: Cursor Set >> Busy|Idle\")"
        n127 = case shown="\"Busy\"" w256 {
          tunnel: w258 -> [w262 w264]
          tunnel: [w261 w263] -> w257
          frame "Idle", Default {
            n128 = call <vilib>:"Unset Busy.vi"("error in (no error)"=w262) -> ("error out"=w261:errorcluster)  [unwired: 10 in]
          }
          frame "Busy" {
            n129 = call <vilib>:"Set Busy.vi"("error in (no error)"=w264) -> ("error out"=w263:errorcluster)  [unwired: 9 in, 1 out]
          }
        }
        n130 = call <vilib>:"Add State(s) to Queue__jki_lib_state_machine.vi"("State(s) in (\"\")"=w260) -> ("States Out"=w259:string)  [unwired: 14 in]
      }
      frame "UI: Front Panel State" {
        # "Argument"
        # "Set Front Panel Open or Closed\n(Usage: \"UI: Front Panel State >> Open|Close\")"
        n131 = Unbundle By Name(w266) -> ("Core.Current VI Reference"=w268:refnum<vi>)
        n132 = case shown="\"Open\", Default" w267 {
          tunnel: w269 -> [w275 w288]
          tunnel: [w277 w289] -> w265
          tunnel: w268 -> [w276 w286]
          frame "Open", Default {
            n133 = property class="VI"(reference=w276, error in=w275) -> (reference out=w273:refnum<vi>, error out=w274:errorcluster, "Front Panel.Open"=w272:bool)
            n134 = case shown="True" w272 {
              tunnel: [w280 w283] -> w277
              tunnel: w274 -> [w279 w283]
              tunnel: w273 -> [w278 _]
              frame False {
                n135 = invoke class="VI" method="FP.Open"(reference=w278, error in=w279, "Activate"=TRUE, "State"=T21."Standard") -> (error out=w280:errorcluster)  [unwired: 1 in, 4 out]
              }
              frame True {
              }
            }
          }
          frame "Close" {
            n136 = property class="VI"(reference=w286, error in=w288) -> (reference out=w285:refnum<vi>, error out=w287:errorcluster, "Front Panel.Open"=w284:bool)
            n137 = case shown="True" w284 {
              tunnel: [w290 w293] -> w289
              tunnel: w287 -> [w290 w292]
              tunnel: w285 -> [_ w291]
              frame False {
              }
              frame True {
                n138 = invoke class="VI" method="FP.Close"(reference=w291, error in=w292) -> (error out=w293:errorcluster)  [unwired: 1 in, 2 out]
              }
            }
          }
        }
        n139 = call <vilib>:"Add State(s) to Queue__jki_lib_state_machine.vi"("State(s) in (\"\")"=w271) -> ("States Out"=w270:string)  [unwired: 14 in]
      }
      frame "---------- Macro ----------" {
        # "Do not put any code in this frame.\n(It is a separator no-op. You can make a copy of this frame to create a new Macro frame)"
        n140 = call <vilib>:"Add State(s) to Queue__jki_lib_state_machine.vi"("State(s) in (\"\")"=w297) -> ("States Out"=w296:string)  [unwired: 14 in]
      }
      frame "Macro: Initialize" {
        w299 = "Data: Initialize\nInitialize Core Data\nUI: Initialize\nUI: Front Panel State >> Open"  # Data: Initialize Initialize Core Data UI: Initialize UI: Front Panel State >> Open
        n141 = call <vilib>:"Add State(s) to Queue__jki_lib_state_machine.vi"("State(s) in Front (\"\")"=w299, "State(s) in (\"\")"=w302) -> ("States Out"=w301:string)  [unwired: 13 in]
      }
      frame "Macro: IV" {
        n142 = call <vilib>:"Add State(s) to Queue__jki_lib_state_machine.vi"("State(s) in Front (\"\")"="4461: SETUP\n4461: CREATE TASKS\n4461: READ WRITE\n4461: FILTER\n4461: PHASE\n4461: LOCKIN\n4461: STOP TASKS", "State(s) in (\"\")"=w307) -> ("States Out"=w306:string)  [unwired: 13 in]
      }
      frame "Macro: Continuous" {
        n143 = case shown="\"Continue\"" w309 {
          tunnel: ["4461: SETUP\n4461: CREATE TASKS\n4461: INFO\n4461: READ WRITE\n4461: FILTER\n4461: PHASE\n4461: LOCKIN" "4461: READ WRITE\n4461: FILTER\n4461: PHASE\n4461: LOCKIN"] -> w308
          frame "Initialize", Default {
          }
          frame "Continue" {
          }
        }
        n144 = call <vilib>:"Add State(s) to Queue__jki_lib_state_machine.vi"("State(s) in Front (\"\")"=w308, "State(s) in (\"\")"=w313) -> ("States Out"=w312:string)  [unwired: 13 in]
      }
      frame "Macro: Exit" {
        w317 = FALSE ("EXIT")
        # "Exit Macro\n(This is called once, when the VI exits)"
        n145 = Unbundle By Name(w316) -> ("Core.Close Panel on Exit?"=w323:bool)
        n146 = local write "EXIT"(w317) -> ()
        n147 = local write "RESET"(w317) -> ()
        n148 = Select(t="UI: Front Panel State >> Close", s=w323, f="") -> (s? t:f=w320:string)
        n149 = call <vilib>:"Add State(s) to Queue__jki_lib_state_machine.vi"("State(s) in (\"\")"=w320, "State(s) at Back (\"\")"="Data: Cleanup\nExit") -> ("States Out"=w318:string)  [unwired: 13 in]
        n150 = call <vilib>:"Add State(s) to Queue__jki_lib_state_machine.vi"("State(s) in Front (\"\")"=w318, "State(s) in (\"\")"=w326) -> ("States Out"=w325:string)  [unwired: 13 in]
      }
      frame "---------- 4461----------" {
        n151 = call <vilib>:"Add State(s) to Queue__jki_lib_state_machine.vi"("State(s) in (\"\")"=w330) -> ("States Out"=w329:string)  [unwired: 14 in]
      }
      frame "4461: INI" {
        n152 = case shown="True" "save config" {
          tunnel: "Instrument" -> [w340 w349]
          tunnel: w334 -> [w347 w352]
          tunnel: [w346 w351] -> w333
          tunnel: "load config" -> [_ w350]
          frame True {
            n153 = local read "AI Configuration"() -> (w343:T17[])
            n154 = local read "AO Configuration"() -> (w344:T16[])
            n155 = local read "DAQ Type"() -> (w345:enum16{"None", "USB 4431", "PXI 446x"})
            n156 = local read "Amplifiers"() -> (w342:enum16{"None", "Krohn Hite", "Femto"})
            n157 = call "config.vi"("Function"=enum16{"write", "read"}."write", "Error In"=w347, "Instrument"=w340, "Amplifiers"=w342, "DAQ Type"=w345, "AO Configuration"=w344, "AI Configuration"=w343) -> ("Error Out"=w346:errorcluster)  [unwired: 4 out]
            n158 = local write "save config"(FALSE ("save config")) -> ()
          }
          frame False {
            n159 = case shown="True" w350 {
              tunnel: w349 -> [_ w354]
              tunnel: w352 -> [w353 w357]
              tunnel: [w353 w356] -> w351
              frame False {
              }
              frame True {
                n160 = local write "load config"(FALSE ("load config")) -> ()
                n161 = call "config.vi"("Function"=enum16{"write", "read"}."read", "Error In"=w357, "Instrument"=w354) -> ("Amplifiers"=w361:enum16{"None", "Krohn Hite", "Femto"}, "DAQ Type"=w362:enum16{"None", "USB 4431", "PXI 446x"}, "AO Configuration 2"=w359:T27, "AI Configuration 2"=w360:T28, "Error Out"=w356:errorcluster)  [unwired: 4 in]
                n162 = local write "AI Configuration"(w360) -> ()
                n163 = local write "AO Configuration"(w359) -> ()
                n164 = local write "DAQ Type"(w362) -> ()
                n165 = local write "Amplifiers"(w361) -> ()
              }
            }
          }
        }
        n166 = call <vilib>:"Add State(s) to Queue__jki_lib_state_machine.vi"("State(s) in (\"\")"=w337, "State(s) at Back (\"\")"="4461: RESET" ("State(s) at Back (\"\")")) -> ("States Out"=w338:string)  [unwired: 13 in]
      }
      frame "4461: SETUP" {
        n167 = case shown="True" "auto size" {
          tunnel: [w377 w397] -> w370
          tunnel: "DAQ Type" -> [_ w394]
          tunnel: w364 -> [w378 w385]
          frame False {
            n168 = Bundle(cluster=cluster{"Fs":i32, "#s":i32} {"Fs"=204000, "#s"=34} ("sampling info"), "Fs"="Fs", "#s"="#s") -> (w376:cluster{"Fs":i32, "#s":i32})
            "sampling info" <- w376
            n169 = Bundle By Name(cluster=w378, "sampling info"=w376, "to"=0) -> (w377:T24)
          }
          frame True {
            # "max Fs"
            n170 = local read "Channels: AO"() -> (w395:T6)
            n171 = Unbundle By Name(w395) -> ("AO f (Hz)"=w393:T9)
            n172 = case shown="\"None\"" w394 {
              tunnel: [102400.0 ("upper limit") 204800.0 ("upper limit") 204800.0 ("upper limit")] -> w384
              frame "USB 4431", Default {
              }
              frame "PXI 446x" {
              }
              frame "None" {
              }
            }
            n173 = Index Array(array=w393) -> (element=w396:dbl)  [unwired: 1 in]
            n174 = Multiply(x="frequency multiplier", y=w396) -> (x*y=w392:dbl)
            n175 = In Range and Coerce(upper limit=w384, x=w392, lower limit=1000.0) -> (coerced(x)=w390:dbl)  [unwired: 1 out]
            n176 = call "Fs and Ns for integer periods.vi"("f_integer"=w396, "Fs"=w390) -> ("#s_integer"=w386:dbl, "Fs_integer"=w388:dbl)  [unwired: 8 in]
            n177 = In Range and Coerce(upper limit=w384, x=w386, lower limit=128.0) -> (coerced(x)=w381:dbl)  [unwired: 1 out]
            n178 = In Range and Coerce(upper limit=w384, x=w388, lower limit=1000.0) -> (coerced(x)=w382:dbl)  [unwired: 1 out]
            n179 = Unbundle By Name(w385) -> ("sampling info"=w399:cluster{"Fs":dbl, "#s":dbl})
            n180 = local write "#s"(w381) -> ()
            n181 = local write "Fs"(w382) -> ()
            n182 = Bundle By Name(cluster=w399, "Fs"=w382, "#s"=w381) -> (w398:cluster{"Fs":dbl, "#s":dbl})
            n183 = Bundle By Name(cluster=w385, "sampling info"=w398, "to"=0) -> (w397:T24)
          }
        }
        n184 = case shown="\"None\"" "DAQ Type" {
          frame "USB 4431", Default {
          }
          frame "PXI 446x" {
          }
          frame "None" {
            n185 = local write "Amplifiers"(enum16{"None", "Krohn Hite", "Femto"}."None" ("Amplifiers")) -> ()
          }
        }
        n186 = case shown="\"USB 4431\"" "DAQ Type" {
          tunnel: [u32 0 u32 0 u32 16448250] -> w368
          tunnel: [u32 6618880 u32 6618880 u32 16711680] -> w367
          frame "USB 4431" {
          }
          frame "PXI 446x" {
          }
          frame "None" {
          }
        }
        n187 = property on="DAQ Type" class="Enum (strict)"() -> ("RingText.Text"=→"DAQ mode string":string)  [unwired: 2 in, 2 out]
        n188 = property on="DAQ mode string" class="Str"("Text.BG Color"=w367, "Text.FG Color"=w368) -> ()  [unwired: 2 in, 2 out]
        n189 = call <vilib>:"Add State(s) to Queue__jki_lib_state_machine.vi"("State(s) in (\"\")"=w372) -> ("States Out"=w371:string)  [unwired: 14 in]
      }
      frame "4461: CALIBRATE" {
        n190 = Unbundle By Name(w414) -> ("AI task"=w415:refnum<k21>[], "AO task"=w416:refnum<k21>[])
        n191 = call "4461 - Cal Info.vi"("error in (no error)"=w413, "Perform Auto Calibration"=TRUE, "Refnum In 2"=w416, "Refnum In"=w415) -> ("error out"=w412:errorcluster, "Cal Info"=w410:T29)  [unwired: 6 in]
        n192 = local write "Cal Info"(w410) -> ()
        n193 = call <vilib>:"Add State(s) to Queue__jki_lib_state_machine.vi"("State(s) in (\"\")"=w418) -> ("States Out"=w417:string)  [unwired: 14 in]
      }
      frame "4461: INFO" {
        n194 = Unbundle By Name(w423) -> ("AI task"=w424:refnum<k21>[], "AO task"=w425:refnum<k21>[])
        n195 = call "4461 - Cal Info.vi"("error in (no error)"=w422, "Perform Auto Calibration"=FALSE, "Refnum In 2"=w425, "Refnum In"=w424) -> ("error out"=w419:errorcluster, "Cal Info"=w420:T29)  [unwired: 6 in]
        n196 = local write "Cal Info"(w420) -> ()
        n197 = call <vilib>:"Add State(s) to Queue__jki_lib_state_machine.vi"("State(s) in (\"\")"=w427) -> ("States Out"=w426:string)  [unwired: 14 in]
      }
      frame "4461: CREATE TASKS" {
        w435 = 10178 items=["Finite Samples"=10178, "Continuous Samples"=10123] ("sample mode")
        w434 = 10123 items=["Finite Samples"=10178, "Continuous Samples"=10123] ("sample mode")
        n198 = local read "AO Configuration"() -> (w439:T16[])
        n199 = local read "Channels: Lockin"() -> (w432:T13)
        n200 = local read "AI Configuration"() -> (w441:T17[])
        n201 = local read "AI Buffer Size (S)"() -> (w446:i32)
        n202 = local read "IV Curve Mode"() -> (w428:bool)
        n203 = Unbundle By Name(w436) -> ("sampling info"=w437:cluster{"Fs":dbl, "#s":dbl})
        n204 = local read "Channels: AO"() -> (w447:T6)
        n205 = local read "DAQ Type"() -> (w431:enum16{"None", "USB 4431", "PXI 446x"})
        n206 = Equal?(x=w431, y=enum16{"None", "USB 4431", "PXI 446x"}."None" ("DAQ Type")) -> (x = y?=w429:bool)
        n207 = Select(t=w435, s=w428, f=w434) -> (s? t:f=w433:i32)
        n208 = case shown="True" w429 {
          tunnel: w441 -> [w461 _]
          tunnel: w439 -> [w460 _]
          tunnel: [w459 w480] -> w445
          tunnel: w437 -> [w458 w477]
          tunnel: [w457 w480] -> w444
          tunnel: w446 -> [w456 _]
          tunnel: [w455 dbl[] [] ("phase log")] -> w440
          tunnel: w447 -> [w454 w478]
          tunnel: w442 -> [w453 w483]
          tunnel: [w452 w482] -> w438
          tunnel: w433 -> [w451 _]
          tunnel: w432 -> [w450 w479]
          tunnel: w428 -> [_ w476]
          frame False {
            n209 = disable-structure shown="Default" {
              disable-tunnel: w461 -> [w473 _]
              disable-tunnel: w460 -> [w472 _]
              disable-tunnel: [w471 _] -> w459
              disable-tunnel: w458 -> [w468 _]
              disable-tunnel: [w470 _] -> w457
              disable-tunnel: w456 -> [w466 _]
              disable-tunnel: [w467 _] -> w455
              disable-tunnel: w454 -> [w469 _]
              disable-tunnel: w453 -> [w465 _]
              disable-tunnel: [w464 _] -> w452
              disable-tunnel: w451 -> [w463 _]
              disable-tunnel: w450 -> [w462 _]
              frame condition #0 (active) {
                n210 = call "4461 - Create IO Channels Parallel Uneven.vi"("sample mode"=w463, "Channels: Lockin"=w462, "error in"=w465, "AI Buffer Size (S)"=w466, "sampling info"=w468, "AO"=w469, "AO Configuration"=w472, "AI Configuration"=w473) -> ("AO Task"=w470:refnum<k21>[], "AI task"=w471:refnum<k21>[], "error out"=w464:errorcluster, "phase log"=w467:dbl[])
              }
              frame condition #1 {
              }
            }
          }
          frame True {
            w480 = refnum<k21>[] [] ("AI task")
            # "simulate mode"
            n211 = Not(x=w476) -> (.not. x?=w475:bool)
            n212 = local read "Gain"() -> (w474:dbl[])
            n213 = call "4461 - Create AO waveforms.vi"("sampling info"=w477, "reset signal"=w475, "AO"=w478) -> ()  [unwired: 5 in, 4 out]
            n214 = call "4461 - Create Reference Waveforms.vi"("sampling info"=w477, "reset signal"=w475, "Lockin"=w479) -> ()  [unwired: 5 in, 4 out]
            n215 = call <userlib>:"FGV - KH Gain.vi"("error in"=w483, "Function"=enum16{"write", "read"}."write", "Gains"=w474) -> ("error out"=w482:errorcluster)  [unwired: 3 in, 1 out]
            n216 = local write "Gain"(w474) -> ()
          }
        }
        n217 = local write "phase log"(w440) -> ()
        n218 = Bundle By Name(cluster=w436, "AI task"=w445, "AO task"=w444) -> (w443:T24)
        n219 = call <vilib>:"Add State(s) to Queue__jki_lib_state_machine.vi"("State(s) in (\"\")"=w449) -> ("States Out"=w448:string)  [unwired: 14 in]
      }
      frame "4461: READ WRITE" {
        n220 = Unbundle By Name(w514) -> ("AI task"=w485:refnum<k21>[], "sampling info"=w498:cluster{"Fs":dbl, "#s":dbl})
        n221 = local read "IV Curve Mode"() -> (w486:bool)
        n222 = local read "..........reset signal"() -> (w488:bool)
        n223 = local read "....measure offset"() -> (w513:bool)
        n224 = local read "Channels: AO"() -> (w507:T6)
        n225 = Unbundle By Name(w507) -> ("AO amp (V)"=w504:T7)
        n226 = Array Size(array=w504) -> (size(s)=w505:i32)
        n227 = Initialize Array(0.0 ("element"), w505) -> (w502:dbl[])
        n228 = local read "Channels: Lockin"() -> (w511:T13)
        n229 = Bundle By Name(cluster=w507, "AO amp (V)"=w502) -> (w506:T6)
        n230 = Get Date/Time In Seconds() -> (seconds since 1Jan1904=w495:timestamp)
        n231 = Format Date/Time String(time format string (%c)="%H:%M:%S%1u   %Y-%m-%d", seconds (now)=w495) -> (date/time string=→"time and date":string)  [unwired: 1 in]
        n232 = Select(t=w506, s=w513, f=w507) -> (s? t:f=w512:T6)
        n233 = Or(x=w486, y=w488) -> (x .or. y?=w487:bool)
        n234 = local read "DAQ Type"() -> (w497:enum16{"None", "USB 4431", "PXI 446x"})
        n235 = call "4461 - Create AO waveforms.vi"("error in (no error)"=w524, "sampling info"=w498, "reset signal"=w487, "AO"=w512) -> ("error out"=w510:errorcluster, "phase out"=w508:dbl[], "AO Array"=w509:waveform(dbl)[])  [unwired: 4 in, 1 out]
        n236 = call "4461 - Create Reference Waveforms.vi"("error in (no error)"=w524, "sampling info"=w498, "reset signal"=w487, "Lockin"=w511) -> ("error out"=w516:errorcluster, "AO Array"=w501:waveform(dbl)[])  [unwired: 4 in, 2 out]
        n237 = call-poly <userlib>:"Empty Array__ogtk.vi"("Array"=w485) -> ("Empty Array?"=w490:bool)  [unwired: 8 in]
        n238 = local write "phase log"(w508) -> ()
        n239 = Equal?(x=w497, y=enum16{"None", "USB 4431", "PXI 446x"}."None" ("DAQ Type")) -> (x = y?=w496:bool)
        n240 = Or(x=w490, y=w496) -> (x .or. y?=w491:bool)
        n241 = case shown="False" w491 {
          tunnel: [w544 w558] -> w499
          tunnel: w509 -> [w534 w556]
          tunnel: w498 -> [w541 w554]
          tunnel: w514 -> [w542 _]
          tunnel: w510 -> [w535 w557]
          tunnel: [w543 w557] -> w523
          tunnel: [w540 w556] -> w500
          tunnel: w486 -> [w539 _]
          frame False {
            n242 = Unbundle By Name(w542) -> ("AI task"=w537:refnum<k21>[], "AO task"=w536:refnum<k21>[])
            n243 = property on="DAQ mode string" class="Str"("Text.BG Color"=u32 6618880) -> ()  [unwired: 2 in, 2 out]
            n244 = disable-structure shown="Default" {
              disable-tunnel: [w546 _] -> w544
              disable-tunnel: w534 -> [w547 w553]
              disable-tunnel: w541 -> [w548 _]
              disable-tunnel: w537 -> [w550 _]
              disable-tunnel: w535 -> [w552 _]
              disable-tunnel: [w551 _] -> w543
              disable-tunnel: [w547 w553] -> w540
              disable-tunnel: w536 -> [w549 _]
              disable-tunnel: w539 -> [w545 _]
              frame condition #0 (active) {
                n245 = call "4461 - AI AND AI - Read AND Write Uneven.vi"("Reset"=w545, "AO Array"=w547, "error in (no error)"=w552, "sampling info"=w548, "AO Task"=w549, "AI task"=w550) -> ("error out"=w551:errorcluster, "Input Signals"=w546:waveform(dbl)[])  [unwired: 4 in]
              }
              frame condition #1 {
              }
            }
          }
          frame True {
            n246 = call "4461 Sim - Noise.vi"("data"=w556, "sampling info"=w554) -> ("Data"=w558:waveform(dbl)[])  [unwired: 5 in]
            n247 = local write "DAQ Type"(enum16{"None", "USB 4431", "PXI 446x"}."None" ("DAQ Type")) -> ()
          }
        }
        n248 = case shown="True" w490 {
          frame False {
          }
          frame True {
            # "flash colors to alert user"
            n249 = property on="DAQ mode string" class="Str"() -> ("Text.BG Color"=w530:u32)  [unwired: 2 in, 2 out]
            n250 = Equal?(x=w530, y=u32 16711680) -> (x = y?=w529:bool)
            n251 = case shown="False" w529 {
              tunnel: [u32 16711680 u32 16448250] -> w528
              frame False {
              }
              frame True {
              }
            }
            n252 = property on="DAQ mode string" class="Str"("Text.BG Color"=w528) -> ()  [unwired: 2 in, 2 out]
          }
        }
        n253 = Index Array(array=w499) -> (element=w521:waveform(dbl))  [unwired: 1 in]
        n254 = local write "time since trigger"(0.0 ("time since trigger")) -> ()
        n255 = Unbundle By Name(w521) -> ("Y"=w520:dbl[])
        n256 = Bundle By Name(cluster=w514, "Input Signals"=w499, "Ouput Signals"=w500, "REF"=w501) -> (w525:T24)
        n257 = call-poly <userlib>:"Empty Array__ogtk.vi"("Array"=w520) -> ("Empty Array?"=w518:bool)  [unwired: 8 in]
        n258 = Merge Errors(w523, w516) -> (w522:errorcluster)
        n259 = Select(t="4461: RESET" ("State(s) at Back (\"\")"), s=w518, f="" ("State(s) at Back (\"\")")) -> (s? t:f=w489:string)
        n260 = call <vilib>:"Add State(s) to Queue__jki_lib_state_machine.vi"("State(s) in Front (\"\")"=w489, "State(s) in (\"\")"=w527) -> ("States Out"=w526:string)  [unwired: 13 in]
      }
      frame "4461: FILTER" {
        w560 = TRUE ("averaging")
        n261 = Unbundle By Name(w565) -> ("Ouput Signals"=w563:waveform(dbl)[], "Input Signals"=w559:waveform(dbl)[], "REF"=w573:waveform(dbl)[])
        n262 = local read "decimating factor"() -> (w561:i32)
        n263 = call "decimate_waveforms.vi"("Input Signal"=w563, "averaging"=w560, "decimating factor"=w561, "error in (no error)"=w578) -> ("Decimated Waveforms"=w562:waveform(dbl)[], "error out"=w577:errorcluster)  [unwired: 5 in]
        n264 = call "decimate_waveforms.vi"("Input Signal"=w559, "averaging"=w560, "decimating factor"=w561, "error in (no error)"=w578) -> ("Decimated Waveforms"=w571:waveform(dbl)[], "error out"=w580:errorcluster)  [unwired: 5 in]
        n265 = call "decimate_waveforms.vi"("Input Signal"=w573, "averaging"=w560, "decimating factor"=w561, "error in (no error)"=w578) -> ("Decimated Waveforms"=w566:waveform(dbl)[], "error out"=w579:errorcluster)  [unwired: 5 in]
        n266 = local read "offsets"() -> (w583:dbl[])
        n267 = Subtract(x=w571, y=w583) -> (x-y=w570:waveform(dbl)[])
        n268 = Merge Errors(w577, w580, w579) -> (w575:errorcluster)
        n269 = case shown="True" "60 Hz prefilter" {
          tunnel: w570 -> [w591 w593]
          tunnel: [w591 w592] -> w569
          frame False {
          }
          frame True {
            n270 = call "Prefilter_60Hz_Notch.vi"("Array"=w593) -> ("Array 2"=w592:waveform(dbl)[])  [unwired: 10 in]
          }
        }
        n271 = local read "............zero offset"() -> (w574:bool)
        n272 = local read "....measure offset"() -> (w576:bool)
        n273 = Index Array(array=w566) -> (element=w582:waveform(dbl))  [unwired: 1 in]
        n274 = case shown="True" "LP prefilter" {
          tunnel: w569 -> [w587 w590]
          tunnel: [w587 w589] -> w568
          tunnel: "LP cutoff (Hz)" -> [_ w588]
          frame False {
          }
          frame True {
            n275 = call "Prefilter_LP.vi"("high cutoff freq [Hz]"=w588, "Array"=w590) -> ("Array 2"=w589:waveform(dbl)[])  [unwired: 9 in]
          }
        }
        n276 = Unbundle By Name(w582) -> ("dt"=w581:dbl)
        n277 = local write "dt"(w581) -> ()
        n278 = case shown="True" w576 {
          tunnel: w565 -> [w600 w605]
          frame False {
            n279 = Unbundle By Name(w600) -> ("Input Signals"=w599:waveform(dbl)[])
            n280 = for {
              tunnel: w599 -> [w602] mode=indexing
              tunnel: [w601] -> w598 mode=indexing
              n281 = call-poly <vilib>:"Mean.vi"("X"=w602) -> ("mean"=w601:dbl)  [unwired: 1 out]
            }
            n282 = local write "mean"(w598) -> ()
          }
          frame True {
            n283 = Unbundle By Name(w605) -> ("Input Signals"=w604:waveform(dbl)[])
            n284 = for {
              tunnel: w604 -> [w607] mode=indexing
              tunnel: [w606] -> w603 mode=indexing
              n285 = call-poly <vilib>:"Mean.vi"("X"=w607) -> ("mean"=w606:dbl)  [unwired: 1 out]
            }
            n286 = local write "offsets"(w603) -> ()
            n287 = local write "mean"(w603) -> ()
          }
        }
        n288 = case shown="False" w574 {
          tunnel: w559 -> [_ w594]
          frame False {
          }
          frame True {
            n289 = Array Size(array=w594) -> (size(s)=w596:i32)
            n290 = Initialize Array(0.0 ("mean"), w596) -> (w595:dbl[])
            n291 = local write "offsets"(w595) -> ()
          }
        }
        n292 = Bundle By Name(cluster=w565, "Ouput Signals"=w562, "Input Signals"=w568, "REF"=w566) -> (w584:T24)
        n293 = call <vilib>:"Add State(s) to Queue__jki_lib_state_machine.vi"("State(s) in (\"\")"=w586) -> ("States Out"=w585:string)  [unwired: 14 in]
      }
      frame "4461: PHASE" {
        n294 = local read "Results\n(X, Y, R, Theta, mean)"() -> (w619:dbl[][])
        n295 = local read "autophase?\n(experimental)"() -> (w618:bool)
        n296 = local read "phase log"() -> (w620:dbl[])
        n297 = local read "Channels: Lockin"() -> (w616:T13)
        n298 = local read "Channels: AO"() -> (w615:T6)
        n299 = call "lockin - Set all f same.vi"("all  frequencies same?"="............all  f same", "Lockin"=w616, "AO"=w615) -> ("Lockin 2"=w613:T22, "AO 2"=w612:T23)  [unwired: 7 in]
        n300 = call "lockin - Set REF phase equals zero.vi"("reset REF phi to zero"="...............reset REF", "Channels: Lockin"=w613, "Channels: AO"=w612) -> ("Channels: Lockin 2"=w608:T22, "Channels: AO 2"=w614:T23)  [unwired: 7 in]
        n301 = case shown="True" w618 {
          tunnel: w620 -> [_ w629]
          tunnel: w619 -> [_ w628]
          tunnel: w608 -> [w624 w626]
          tunnel: [w624 w625] -> w609
          frame False {
          }
          frame True {
            # "do this for EACH lockin...\n- replace PID array with PID SV\n-  advance \"results\" by 8?\n- this should go BEFORE REF\nwaveform is generated"
            n302 = Index Array(array=w628, index (col)=3 ("index (row)")) -> (element=w631:dbl[])  [unwired: 1 in]
            n303 = call "Simple PID Array.vi"("D"="D", "I"="I", "P"="P", "process variable"=w631) -> ("output value"=w635:dbl[])  [unwired: 7 in]
            n304 = Subtract(x=w629, y=w635) -> (x-y=w627:dbl[])
            n305 = Bundle By Name(cluster=w626, "REF phi (deg)"=w627) -> (w625:T22)
          }
        }
        n306 = local write "Channels: AO"(w614) -> ()
        n307 = local write "Channels: Lockin"(w609) -> ()
        n308 = call <vilib>:"Add State(s) to Queue__jki_lib_state_machine.vi"("State(s) in (\"\")"=w623) -> ("States Out"=w622:string)  [unwired: 14 in]
      }
      frame "4461: LOCKIN" {
        # "Display stuff and lockin calculations"
        n309 = Unbundle By Name(w686) -> ("Ouput Signals"=w654:waveform(dbl)[], "Input Signals"=w643:waveform(dbl)[], "REF"=w653:waveform(dbl)[], "sampling info"=w660:cluster{"Fs":dbl, "#s":dbl})
        n310 = local read "TC (s)"() -> (w649:dbl)
        n311 = local read "mean"() -> (w679:dbl[])
        n312 = local read "order"() -> (w684:i32)
        n313 = local read "Gain"() -> (w658:dbl[])
        n314 = local read "Gain"() -> (w636:dbl[])
        n315 = Select(t="applied signals (V)" ("Y Scale.Name Label.Text"), s="Output signals?", f="REF signal (arb)" ("Y Scale.Name Label.Text")) -> (s? t:f=w659:string)
        n316 = Select(t=w654, s="Output signals?", f=w653) -> (s? t:f=w666:waveform(dbl)[])
        n317 = Divide(x=w643, y=w636) -> (x/y=w656:waveform(dbl)[])
        n318 = property on="Reference Graph" class="WFGraph (strict)"("YScale.NameLbl.Text"=w659) -> ()  [unwired: 2 in, 2 out]
        n319 = Divide(x=w679, y=w658) -> (x/y=w678:dbl[])
        n320 = call "Display n or dt.vi"("Display n?"="Display n?", "Input Waveforms"=w643) -> ("Output Waveforms"=w673:waveform(dbl)[])  [unwired: 9 in]
        n321 = call "Display n or dt.vi"("Display n?"="Display n?", "Input Waveforms"=w666) -> ("Output Waveforms"=w671:waveform(dbl)[])  [unwired: 9 in]
        n322 = call "decimate_waveforms.vi"("Input Signal"=w671, "averaging"=FALSE, "decimating factor"="decimate graph") -> ("Decimated Waveforms"=→"Reference Graph":waveform(dbl)[])  [unwired: 6 in, 1 out]
        n323 = call "decimate_waveforms.vi"("Input Signal"=w673, "averaging"=FALSE, "decimating factor"="decimate graph") -> ("Decimated Waveforms"=→"Signals Graph":waveform(dbl)[])  [unwired: 6 in, 1 out]
        n324 = call "4461 - Lockin Engine.vi"("order"=w684, "TC (s)"=w649, "sampling info"=w660, "Reference In"=w653, "Signal in"=w656) -> ("filter fC (Hz)"=w664:dbl, "Results (X,Y,R,Theta)"=w681:dbl[][])  [unwired: 5 in]
        n325 = Transpose 2D Array(2D array=w681) -> (transposed array=w677:dbl[][])
        n326 = Build Array (concatenate)(w677, w678) -> (w680:dbl[][])
        n327 = Index Array(array=w656) -> (element=w667:waveform(dbl))  [unwired: 1 in]
        n328 = call "FGV - Signals - Output.vi"("Function"=enum16{"write", "read"}."write", "input signal"=w654) -> ()  [unwired: 4 in, 2 out]
        n329 = call "FGV - Signals - Input.vi"("Function"=enum16{"write", "read"}."write", "input signal"=w656) -> ()  [unwired: 4 in, 2 out]
        n330 = local read "Channel"() -> (w665:dbl)
        n331 = local write "filter fC (Hz)"(w664) -> ()
        n332 = local read "Display"() -> (w683:enum16{"X and Y", "R and Theta"})
        n333 = Transpose 2D Array(2D array=w680) -> (transposed array=w670:dbl[][])
        "Results\n(X, Y, R, Theta, mean)" <- w670
        n334 = Unbundle By Name(w667) -> ("t0"=w655:timestamp)
        n335 = Array Size(array=w643) -> (size(s)=w642:i32)
        n336 = Array Size(array=w636) -> (size(s)=w641:i32)
        n337 = call "format display.vi"("Channel"=w665, "Display"=w683, "Results (X,Y,R,Theta)"=w681, "t0"=w655) -> ("X/R"=→"X or R":dbl, "Array 2"=→"XY Graph":cluster{dbl[], dbl[]}[], "Y/Theta Array"=→"Display Y (or Theta)":waveform(dbl)[], "X/R Array"=→"Display X (or R)":waveform(dbl)[], "Y/R"=→"Y or Theta":dbl)  [unwired: 3 in]
        n338 = local read "Tab Control 2"() -> (w645:T1)
        n339 = Greater?(x=w642, y=w641) -> (0:w640:bool)
        n340 = call "FGV - Lockin Results.vi"("Function"=enum16{"write", "read"}."write", "Input Signals"=w670) -> ()  [unwired: 4 in, 2 out]
        n341 = case shown="False" w640 {
          tunnel: [w691 "Check Chan#" ("DAQ mode string")] -> w639
          tunnel: [u32 6618880 u32 16711680] -> w638
          tunnel: [u32 0 u32 16448250] -> w637
          frame False {
            n342 = property on="DAQ Type" class="Enum (strict)"() -> ("RingText.Text"=w691:string)  [unwired: 2 in, 2 out]
          }
          frame True {
          }
        }
        n343 = case shown="\"PS\"" w645 {
          tunnel: ["" ("State(s) at Back (\"\")") "4461: FFT" ("State(s) at Back (\"\")")] -> w644
          frame Default {
          }
          frame "PS" {
          }
        }
        n344 = local write "DAQ mode string"(w639) -> ()
        n345 = property on="DAQ mode string" class="Str"("Text.BG Color"=w638, "Text.FG Color"=w637) -> ()  [unwired: 2 in, 2 out]
        n346 = call <vilib>:"Add State(s) to Queue__jki_lib_state_machine.vi"("State(s) in Front (\"\")"=w644, "State(s) in (\"\")"=w688) -> ("States Out"=w685:string)  [unwired: 13 in]
      }
      frame "4461: FFT" {
        n347 = Unbundle By Name(w717) -> ("Input Signals"=w699:waveform(dbl)[])
        n348 = local read "Gain"() -> (w715:dbl[])
        n349 = Divide(x=w699, y=w715) -> (x/y=w706:waveform(dbl)[])
        n350 = call-poly <vilib>:"FFT Power Spectrum and PSD.vi"("window parameter"="window parameter", "export mode"="export mode", "averaging parameters"="averaging parameters", "restart averaging (F)"="restart averaging (F)", "dB On (F)"=TRUE, "window"="window", "time signals"=w706) -> ("averages completed"=→"averages\ncompleted":dbl, "averaging done"=→"averaging done":bool, "Power Spectrum / PSD"=w697:cluster{"f0":dbl, "df":dbl, "magnitude":dbl[]}[])  [unwired: 1 in, 1 out]
        "PS dB" <- w697
        n351 = for {
          tunnel: w697 -> [w737] mode=indexing
          tunnel: [w732] -> w698 mode=indexing
          n352 = Unbundle By Name(w737) -> ("df"=w739:dbl, "magnitude"=w738:dbl[])  [unwired: 1 out]
          n353 = Bundle By Name("dt"=w739, "Y"=w738) -> (w736:waveform(dbl))  [unwired: 1 in]
          n354 = call-poly <vilib>:"Waveform to XY Pairs.vi"("waveform in"=w736) -> ("XY pairs"=w735:cluster{"x":timestamp, "y":dbl}[])  [unwired: 8 in, 2 out]
          n355 = for {
            tunnel: w735 -> [w743] mode=indexing
            tunnel: [w741] -> w733 mode=indexing
            tunnel: [w740] -> w734 mode=indexing
            n356 = Unbundle(w743) -> ("x"=w742:timestamp, "y"=w741:dbl)
            n357 = To Double Precision Float(number=w742) -> (double precision float=w740:dbl)
          }
          n358 = Bundle(w734, w733) -> (w732:cluster{dbl[], dbl[]})  [unwired: 1 in]
        }
        n359 = property on="PS dB" class="WFGraph (strict)"("Active Cursor"=u32 1) -> ("Cursor.Cursor X"=w711:dbl)  [unwired: 2 in, 2 out]
        n360 = property on="PS dB" class="WFGraph (strict)"("Active Cursor"=u32 0) -> ("Cursor.Cursor X"=w712:dbl)  [unwired: 2 in, 2 out]
        n361 = Build Array(w712, w711) -> (w710:dbl[])
        n362 = for {
          tunnel: w698 -> [w731] mode=indexing
          tunnel: w710 -> [w730]
          tunnel: [w722] -> w709 mode=indexing
          n363 = Array Max & Min(array=w730) -> (max value=w729:dbl, min value=w727:dbl)  [unwired: 2 out]
          n364 = Unbundle(w731) -> (w728:dbl[], w726:dbl[])
          n365 = Threshold 1D Array(2:w729, 3:w728) -> (0:w725:dbl)  [unwired: 1 in]
          n366 = Threshold 1D Array(2:w727, 3:w728) -> (0:w724:dbl)  [unwired: 1 in]
          n367 = Subtract(x=w725, y=w724) -> (x-y=w723:dbl)
          n368 = Array Subset(array=w726, index=w724, length=w723) -> (w721:dbl[])
          n369 = Add Array Elements(numeric array=w721) -> (sum=w722:dbl)
        }
        n370 = Build Array(w709) -> (→"PS Chart":dbl[][])
        n371 = call <vilib>:"Add State(s) to Queue__jki_lib_state_machine.vi"("State(s) in (\"\")"=w720) -> ("States Out"=w718:string)  [unwired: 14 in]
      }
      frame "4461: SAVE" {
        w746 = "FFT" ("filename")
        w745 = "signal" ("filename")
        # "Wait for Trigger signal from other VI"
        n372 = local read "PS dB"() -> (w762:cluster{"f0":dbl, "df":dbl, "magnitude":dbl[]}[])
        n373 = Get Date/Time In Seconds() -> (seconds since 1Jan1904=w753:timestamp)
        n374 = local read "Path"() -> (w744:path)
        n375 = for {
          tunnel: w762 -> [w782] mode=indexing
          tunnel: [w777] -> w757 mode=indexing
          n376 = Unbundle By Name(w782) -> ("df"=w784:dbl, "magnitude"=w783:dbl[])  [unwired: 1 out]
          n377 = Bundle By Name("dt"=w784, "Y"=w783) -> (w781:waveform(dbl))  [unwired: 1 in]
          n378 = call-poly <vilib>:"Waveform to XY Pairs.vi"("waveform in"=w781) -> ("XY pairs"=w780:cluster{"x":timestamp, "y":dbl}[])  [unwired: 8 in, 2 out]
          n379 = for {
            tunnel: w780 -> [w788] mode=indexing
            tunnel: [w786] -> w778 mode=indexing
            tunnel: [w785] -> w779 mode=indexing
            n380 = Unbundle(w788) -> ("x"=w787:timestamp, "y"=w786:dbl)
            n381 = To Double Precision Float(number=w787) -> (double precision float=w785:dbl)
          }
          n382 = Bundle(w779, w778) -> (w777:cluster{dbl[], dbl[]})  [unwired: 1 in]
        }
        n383 = call "FGV - Signals - Input.vi"("error in"=w754, "Function"=enum16{"write", "read"}."read") -> ("error out"=w755:errorcluster, "input signal"=w761:waveform(dbl)[])  [unwired: 4 in]
        n384 = for {
          tunnel: [w769] -> w760 mode=indexing
          tunnel: w761 -> [w768] mode=indexing
          n385 = call-poly <vilib>:"Waveform to XY Pairs.vi"("waveform in"=w768) -> ("XY pairs"=w772:cluster{"x":timestamp, "y":dbl}[])  [unwired: 8 in, 2 out]
          n386 = for {
            tunnel: w772 -> [w776] mode=indexing
            tunnel: [w774] -> w770 mode=indexing
            tunnel: [w773] -> w771 mode=indexing
            n387 = Unbundle(w776) -> ("x"=w775:timestamp, "y"=w774:dbl)
            n388 = To Double Precision Float(number=w775) -> (double precision float=w773:dbl)
          }
          n389 = Bundle(w771, w770) -> (w769:cluster{dbl[], dbl[]})  [unwired: 1 in]
        }
        n390 = Format Date/Time String(time format string (%c)="%Y-%m-%d", seconds (now)=w753) -> (date/time string=w751:string)  [unwired: 1 in]
        n391 = Build Path(base path=w744, name or relative path=w751) -> (appended path=w749:path)
        n392 = Build Path(base path=w749, name or relative path=w745) -> (appended path=w748:path)
        n393 = call <userlib>:"LV to ITX XY AutoPlot.vi"("filename"=w745, "path"=w748, "Notes"="Notes", "XY Array"=w760, "wavenames (.Vx, etc)"=string[] ["ch0", "ch1", "ch2", "ch3", "ch4", "ch5", "ch6", "ch7"]) -> ()  [unwired: 10 in, 1 out]
        n394 = Build Path(base path=w749, name or relative path=w746) -> (appended path=w747:path)
        n395 = local write "Save Data"(FALSE ("SAVE DATA")) -> ()
        n396 = call <userlib>:"LV to ITX XY AutoPlot.vi"("filename"=w746, "path"=w747, "Notes"="Notes", "XY Array"=w757, "wavenames (.Vx, etc)"=string[] ["FFT0", "FFT1", "FFT2", "FFT3", "FFT4", "FFT5", "FFT6", "FFT7"], "X,Y Log"=i32[] [1, 1]) -> ()  [unwired: 9 in, 1 out]
        n397 = call <vilib>:"Add State(s) to Queue__jki_lib_state_machine.vi"("State(s) in (\"\")"=w767) -> ("States Out"=w766:string)  [unwired: 14 in]
      }
      frame "4461: STOP TASKS" {
        w791 = refnum<k21>[] [] ("AI task")
        w789 = FALSE ("Trigger")
        n398 = Unbundle By Name(w793) -> ("AI task"=w802:refnum<k21>[], "AO task"=w805:refnum<k21>[])
        n399 = local read "DAQ Type"() -> (w799:enum16{"None", "USB 4431", "PXI 446x"})
        n400 = call-poly <userlib>:"Empty Array__ogtk.vi"("Array"=w802) -> ("Empty Array?"=w801:bool)  [unwired: 8 in]
        n401 = Equal?(x=w799, y=enum16{"None", "USB 4431", "PXI 446x"}."None" ("DAQ Type")) -> (x = y?=w798:bool)
        n402 = Or(x=w798, y=w801) -> (x .or. y?=w800:bool)
        n403 = case shown="False" w800 {
          tunnel: w805 -> [w809 _]
          tunnel: w803 -> [w808 w837]
          tunnel: [w807 w837] -> w795
          tunnel: w802 -> [w806 _]
          frame False {
            n404 = disable-structure shown="Default" {
              disable-tunnel: w809 -> [w811 _]
              disable-tunnel: w808 -> [w812 _]
              disable-tunnel: [w813 _] -> w807
              disable-tunnel: w806 -> [w810 _]
              frame condition #0 (active) {
                n405 = for {
                  tunnel: w811 -> [w836] mode=indexing
                  tunnel: [w834] -> w818 mode=indexing
                  tunnel: w812 -> [w833]
                  tunnel: [w832] -> w815
                  n406 = call <vilib>:"DAQmx Stop Task.vi"("task/channels in"=w836, "error in"=w833) -> ("task out"=w834:refnum<k21>, "error out"=w832:errorcluster)  [unwired: 12 in]
                  n407 = Wait (ms)(milliseconds to wait=u32 50) -> ()  [unwired: 1 out]
                }
                n408 = for {
                  tunnel: w810 -> [w831] mode=indexing
                  tunnel: [w829] -> w814 mode=indexing
                  tunnel: w815 -> [w828]
                  tunnel: [w827] -> w817
                  n409 = call <vilib>:"DAQmx Stop Task.vi"("task/channels in"=w831, "error in"=w828) -> ("task out"=w829:refnum<k21>, "error out"=w827:errorcluster)  [unwired: 12 in]
                  n410 = Wait (ms)(milliseconds to wait=u32 50) -> ()  [unwired: 1 out]
                }
                n411 = for {
                  tunnel: w818 -> [w826] mode=indexing
                  tunnel: w817 -> [w824]
                  tunnel: [w823] -> w816
                  n412 = call <vilib>:"DAQmx Clear Task.vi"("task in"=w826, "error in"=w824) -> ("error out"=w823:errorcluster)  [unwired: 13 in]
                  n413 = Wait (ms)(milliseconds to wait=u32 50) -> ()  [unwired: 1 out]
                }
                n414 = for {
                  tunnel: w814 -> [w822] mode=indexing
                  tunnel: w816 -> [w820]
                  tunnel: [w819] -> w813
                  n415 = call <vilib>:"DAQmx Clear Task.vi"("task in"=w822, "error in"=w820) -> ("error out"=w819:errorcluster)  [unwired: 13 in]
                  n416 = Wait (ms)(milliseconds to wait=u32 50) -> ()  [unwired: 1 out]
                }
              }
              frame condition #1 {
              }
            }
          }
          frame True {
          }
        }
        n417 = local write "RESET"(w789) -> ()
        n418 = local write "Trigger"(w789) -> ()
        n419 = Bundle By Name(cluster=w793, "AI task"=w791, "AO task"=w791) -> (w792:T24)
        n420 = call <vilib>:"Add State(s) to Queue__jki_lib_state_machine.vi"("State(s) in (\"\")"=w804) -> ("States Out"=w790:string)  [unwired: 14 in]
        n421 = call "FGV - Trigger.vi"("error in"=w795, "Function"=enum16{"write", "read"}."write", "Trigger"=w789) -> ("error out"=w794:errorcluster)  [unwired: 3 in, 1 out]
      }
      frame "4461: RESET" {
        n422 = call <vilib>:"Add State(s) to Queue__jki_lib_state_machine.vi"("State(s) in Front (\"\")"="4461: STOP TASKS", "State(s) in (\"\")"=w842) -> ("States Out"=w838:string)  [unwired: 13 in]
      }
    }
    n423 = call "StateHistory.vi"("Current State in"=w5) -> ("Current State out"=→"Current State":string, "delimited string"=→"State History":string)  [unwired: 9 in]
  }
